vi "EncoderA(D13B)andLoadCell.vi"() -> ()   [LabVIEW 2021]
uses:
  BISS_1SL_interface_7.7.0/lv_interface/enum/BISS_InterfaceEnum.ctl
  BISS_1SL_interface_7.7.0/lv_interface/enum/BISS_InterfaceInfoEnum.ctl
  BISS_1SL_interface_7.7.0/lv_interface/enum/BISS_ComParamEnum.ctl
  BISS_1SL_interface_7.7.0/lv_interface/enum/BISS_FrameParamEnum.ctl
  BISS_1SL_interface_7.7.0/lv_interface/enum/BISS_EdsParamEnum.ctl
  BISS_1SL_interface_7.7.0/lv_interface/enum/BISS_ErrorTypeEnum.ctl
  BISS_1SL_interface_7.7.0/lv_interface/dll_demo/BiSS Interface Demo Functions.ctl
  BISS_1SL_interface_7.7.0/lv_interface/BISS1SL_Interface.lvlib
panel:
  in  "Stop Button":bool
  in  "TabControl":T1(tab)
  in  "BISS_InterfaceInfoEnum":T2 format="0x%02x"
  out "BISS_InterfaceEnum":T3 format="0x%02x"
  in  "BISS_InterfaceEnum":T3=enum."BISS_MB5U" format="0x%02x"
  in  "Close":bool caption="BiSS_Close"
  in  "Get Interface":bool caption="BiSS_GetInterface"
  in  "Set Interface":bool caption="BiSS_SetInterface"
  in  "Open":bool caption="BiSS_Open"
  in  "pcInterfaceOption":string="D13B"
  in  "Get Interface Info":bool caption="BiSS_GetInterfaceInfo"
  out "pcInterfaceInfo":string
  in  "Write Master Params":bool caption="BiSS_WriteMasterParams"
  in  "pcFilename":path
  in  "Load DLL Config":bool caption="BiSS_LoadDLLConfig"
  in  "pcFilename 2":path=path "C:/Users/TSSW/Documents/Kenneth Feb/BISS Test Vi/BiSS_config.cfg"
  in  "Save DLL Config":bool caption="BiSS_SaveDLLConfig"
  in  "Get Slave Label":bool caption="BiSS_GetSlaveLabel"
  in  "ulSlave 2":u32 format="%.0x"
  out "pcCompleteLabel 2":string
  out "pcSlaveLabel 2":string
  out "pcManufacturerLabel 2":string
  in  "Set FTDI Freq":bool caption="BiSS_SetFTDIFreq"
  in  "ulFreqL":u32=4 format="%0x"
  in  "ulFreqH":u32=4 format="%0x"
  out "Force vs Displacement":cluster{"X":dbl, "Y":dbl}[](graph)
  out "Displacement vs Time":waveform(sgl)(graph)
  out "pulValues":u64[](array[numeric]) format="%.0x"
  in  "ulCycleCount":u32 format="%.0x"
  in  "ulContentIndex":u32 format="%.0x"
  in  "ulDataChannel":u32 format="%.0x"
  in  "Get SCD Frame Content Ex":bool caption="BiSS_GetScdFrameContentEx"
  in  "Read SCD Frames":bool caption="BiSS_ReadScdFrames"
  in  "ulCycleCnt":u32=1 format="%.0x"
  out "pulDataScdH":u32[](array[numeric]) format="%.0x"
  out "pulDataScdL":sgl[](array[numeric]) format="%#_8g mm"
  out "pulStatus":u32[](array[numeric]) format="%.0x"
  out "pulTimestamp":u32[](array[numeric]) format="%.0x"
  in  "Get SCD Frame":bool caption="BiSS_GetScdFrame"
  in  "ulFrameIndex":u32 format="%.0x"
  out "pulDataScdH":u32[](array[numeric]) format="%.0x"
  out "pulDataScdL":u32[](array[numeric]) format="%.0x"
  out "pulStatus":u32 format="%.0x"
  out "pulTimestamp":u32 format="%.0x"
  in  "ulDataChannel":u32 format="%.0x"
  in  "Get SCD Frame Ex":bool caption="BiSS_GetScdFrameEx"
  in  "ulCycleCount":u32 format="%.0x"
  out "pulTimestamp":u32[](array[numeric]) format="%.0x"
  out "pulDataScdH":u32[](array[numeric]) format="%.0x"
  out "pulDataScdL":u32[](array[numeric]) format="%.0x"
  out "pulStatus":u32[](array[numeric]) format="%.0x"
  in  "Get SCD Frame Content":bool caption="BiSS_GetScdFrameContent"
  in  "ulDataChannel":u32 format="%.0x"
  in  "ulContentIndex":u32 format="%.0x"
  out "pulValues":u32[](array[numeric]) format="%.0x"
  in  "ulCycleCount":u32 format="%.0x"
  in  "stop":bool
  out "Loop Time [ms]":u32
  in  "Update Time [ms]":u32=1000
  out "error out 2":errorcluster
  in  "data":dbl[](array[numeric])=[0.0] min=0.0 max=7.0 step=0.1
  out "Load Cells Display":string
  out "error out":errorcluster
  out "Load A [kN]":dbl(slide) scale=-100.0..100.0
  out "Load B [kN]":dbl(slide) scale=-60.0..60.0
  out "Load A vs Time":waveform(dbl)(graph)
  out "BISS_ErrorTypeEnum":T4 format="0x%02x"
  in  "Get DLL Version":bool caption="BiSS_GetDLLVersion"
  out "pulDllVersion":u32[](array[numeric]) format="%.0x"
  in  "Calculate CRC":bool caption="BiSS_CalculateCRC"
  in  "ulCrcPoly":u32 format="%.0x"
  in  "pulData":u32[](array[numeric]) format="%.0x"
  in  "ulByteCount":u32 format="%.0x"
  out "pulCheckSum":u32 format="%.0x"
  in  "Calculate CRC Ex":bool caption="BiSS_CalculateCRCEx"
  out "pulCheckSum":u32 format="%.0x"
  in  "ulByteCount":u32 format="%.0x"
  in  "pulData":u32[](array[numeric]) format="%.0x"
  in  "ulCrcPoly":u32 format="%.0x"
  in  "ulCRCStartValue":u32 format="%.0x"
  in  "Get Last Error":bool caption="BiSS_GetLastError"
  out "pulLastError":u32 format="%0x"
  out "pcErrorText":string
  in  "Get MB3U Pins":bool caption="BiSS_GetMB3UPins"
  out "pulDir":u32 format="%.0x"
  out "pulValue":u32 format="%.0x"
  in  "ulDir":u32 format="%.0x"
  in  "Set MB3U Pins":bool caption="BiSS_SetMB3UPins"
  in  "ulValue":u32 format="%.0x"
  in  "Set Slave Label":bool caption="BiSS_SetSlaveLabel"
  in  "ulSlave":u32 format="%.0x"
  in  "pcSlaveLabel":string
  in  "pcManufacturerLabel":string
  in  "pcCompleteLabel":string
  in  "Set SCD Content Labels":bool caption="BiSS_SetScdContentLabels"
  in  "ulDataChannel":u32 format="%.0x"
  in  "ulContentIndex":u32 format="%.0x"
  in  "pcScdContentLabel":string
  in  "pcScdContentUnit":string
  in  "Get SCD Content Labels":bool caption="BiSS_GetScdContentLabels"
  in  "ulDataChannel":u32 format="%.0x"
  in  "ulContentIndex":u32 format="%.0x"
  out "pcSCDContentLabel":string
  out "pcSCDContentUnit":string
  in  "BISS_FrameParamEnum":T5 format="0x%02x"
  in  "BISS_FrameParamEnum":T5 format="0x%02x"
  in  "BISS_ComParamEnum":T6 format="0x%02x"
  in  "BISS_ComParamEnum":T6 format="0x%02x"
  in  "pcFilename":path
  in  "Set Com Param":bool caption="BiSS_SetComParam"
  in  "Auto Detection":bool caption="BiSS_Autodetection"
  in  "ulWriteMasterParams":u32 format="%.0x"
  out "pulSlaveCount":u32 format="%.0x"
  in  "ulValue":u32 format="%.0x"
  in  "Get Com Param":bool caption="BiSS_GetComParam"
  out "pulValue":u32 format="%.0x"
  in  "Set Frame Param":bool caption="BiSS_FrameParamEnum"
  in  "ulDataChannel":u32 format="%.0x"
  in  "ulValue":u32 format="%.0x"
  in  "Get Frame Param":bool caption="BiSS_GetFrameParam"
  out "pulValue":u32 format="%.0x"
  in  "ulDataChannel":u32 format="%.0x"
  in  "Init BiSS Comm":bool caption="BiSS_InitBissComm"
  in  "Write Slave Register":bool caption="BiSS_WriteSlaveRegister"
  in  "ulProtocol":u32 format="%.0x"
  in  "ulSlaveId":u32 format="%.0x"
  in  "ulRegisterAddress":u32 format="%.0x"
  in  "pulRegisterContent":u32[](array[numeric]) format="%.0x"
  in  "pulNumberOfBytes":u32 format="%.0x"
  in  "Read Slave Register":bool caption="BiSS_ReadSlaveRegister"
  in  "ulProtocol":u32 format="%.0x"
  in  "ulSlaveId":u32 format="%.0x"
  in  "ulRegisterAddress":u32 format="%.0x"
  in  "pulNumberOfBytes":u32 format="%.0x"
  out "pulRegisterContent":u32[](array[numeric]) format="%.0x"
  in  "Read SCD":bool caption="BiSS_ReadSCD"
  in  "ulStartControlFrame":u32 format="%.0x"
  out "pulScdValid":u32 format="%.0x"
  out "pulControlFrameEnd":u32 format="%.0x"
  out "pulDataScdH":u32[](array[numeric]) format="%.0x"
  out "pulDataScdL":u32[](array[numeric]) format="%.0x"
  in  "ulIds":u32 format="%.0x"
  in  "ulCmd":u32 format="%.0x"
  in  "Send Command":bool caption="BiSS_SendCommand"
  in  "Get SCD Content":bool caption="BiSS_GetScdContent"
  in  "ulDataChannel":u32 format="%.0x"
  out "pulScdContentValues":u32[](array[numeric]) format="%.0x"
  in  "Get SCD Content Ex":bool caption="BiSS_GetScdContentEx"
  in  "ulDataChannel":u32 format="%.0x"
  out "pulScdContentValues":u64[](array[numeric]) format="%.0x"
  in  "Set SCD Content Params":bool caption="BiSS_SetScdContentParams"
  in  "ulDataChannel":u32 format="%.0x"
  in  "ulContentIndex":u32 format="%.0x"
  in  "pScdContentItems":T7 {"lOffset" format="%.0x"; "ulResolution" format="%.0x"; "ulDataLength" format="%.0x"; "ulZero" format="%.0x"}
  in  "Get SCD Content Params":bool caption="BiSS_GetScdContentParams"
  in  "ulDataChannel":u32 format="%.0x"
  in  "ulContentIndex":u32 format="%.0x"
  out "pScdContentItems":T7 {"ulZero" format="%.0x"; "ulDataLength" format="%.0x"; "ulResolution" format="%.0x"; "lOffset" format="%.0x"}
  in  "BISS_EdsParamEnum":T8 format="0x%02x"
  in  "BISS_EdsParamEnum":T8 format="0x%02x"
  in  "Set EDS Param":bool caption="BiSS_SetEdsParam"
  in  "ulValue":u32 format="%.0x"
  out "pulValue":u32 format="%.0x"
  in  "Get EDS Param":bool caption="BiSS_GetEdsParam"
  in  "Set EDS Register":bool caption="BiSS_SetEdsRegister"
  in  "ulAdr":u32 format="%.0x"
  in  "ulValue":u32 format="%.0x"
  in  "Get EDS Register":bool caption="BiSS_GetEdsRegister"
  in  "ulAdr":u32 format="%.0x"
  out "pulValue":u32 format="%.0x"
  in  "Read EDS Params":bool caption="BiSS_ReadEdsParams"
  in  "ulSlaveId":u32 format="%.0x"
  in  "Write EDS Params":bool caption="BiSS_WriteEdsParams"
  in  "ulSlaveId":u32 format="%.0x"
  in  "pcFilename":path
  in  "Write Master Register":bool caption="BiSS_ WriteMasterRegister"
  in  "ulRegisterAddress":u32 format="%.0x"
  in  "ulRegisterContent":u32 format="%.0x"
  in  "Read Master Register":bool caption="BiSS_ ReadMasterRegister"
  in  "ulRegisterAddress":u32 format="%.0x"
  out "pulRegisterContent":u32 format="%.0x"
  in  "Get Master Register":bool caption="BiSS_ GetMasterRegister"
  in  "ulRegisterAddress":u32 format="%.0x"
  out "pulRegisterContent":u32 format="%.0x"
  in  "Save Master Config":bool caption="BiSS_ SaveMasterConfig"
  in  "pcFilename":path
  in  "Save Register":bool caption="BiSS_ SaveRegister"
  in  "pcFilename":path
  in  "ulStartAdr":u32 format="%.0x"
  in  "ulNumberOfBytes":u32 format="%.0x"
  in  "pulData":u32[](array[numeric]) format="%.0x"
  in  "Load Register":bool caption="BiSS_ LoadRegister"
  in  "ulStartAdr":u32 format="%.0x"
  in  "ulNumberOfBytes":u32 format="%.0x"
  out "pulData":u32[](array[numeric]) format="%.0x"
  # "BiSS Interface Library Demo"
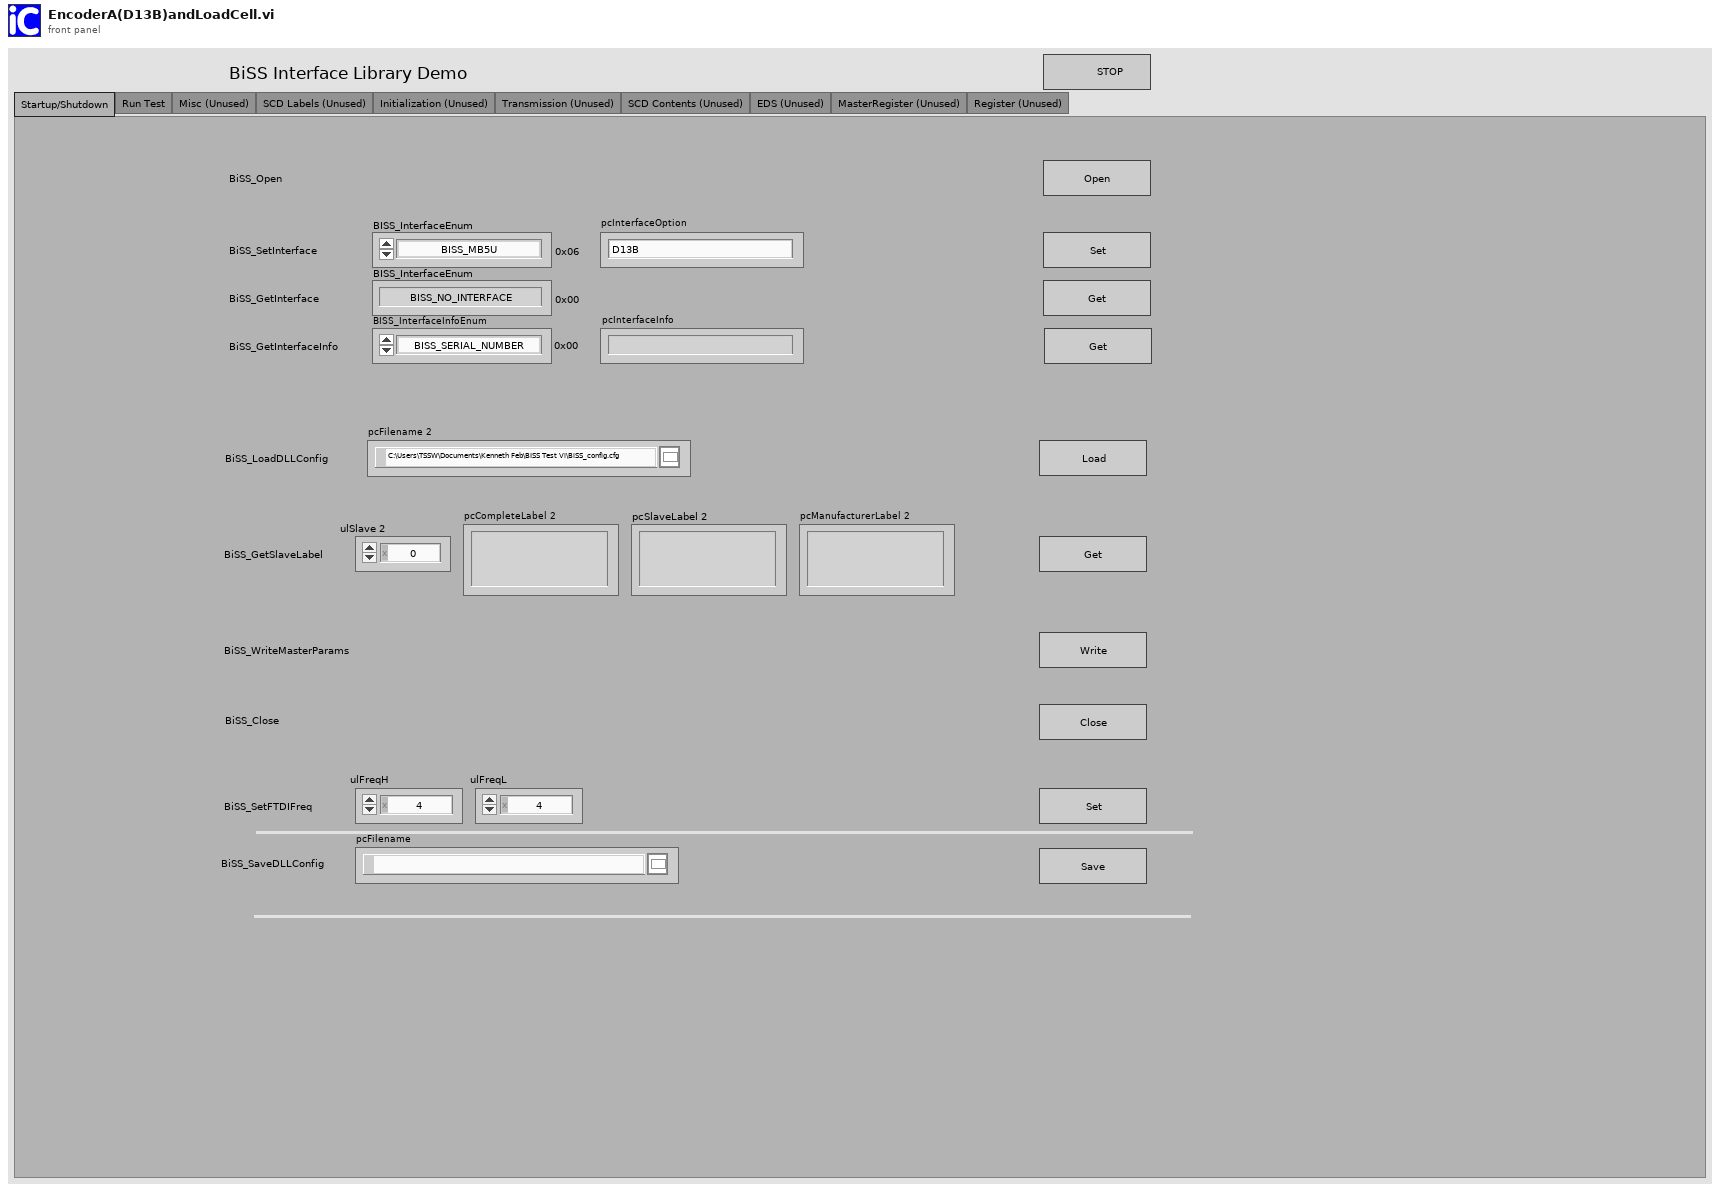
[diagram p1: front panel]
types:
  T1 = enum32{"Startup/Shutdown", "Run Test", "Misc (Unused)", "SCD Labels (Unused)", "Initialization (Unused)", "Transmission (Unused)", "SCD Contents (Unused)", "EDS (Unused)", "MasterRegister (Unused)", "Register (Unused)"}
  T2 = typedef "BISS1SL_Interface.lvlib/BISS_InterfaceInfoEnum.ctl" = enum32{"BISS_SERIAL_NUMBER", "BISS_DRIVER_VERSION"}
  T3 = typedef "BISS1SL_Interface.lvlib/BISS_InterfaceEnum.ctl" = enum32{"BISS_NO_INTERFACE", "BISS_MB3D_INT", "BISS_MB3D_MOT", "BISS_MB3A", "BISS_MB3U", "BISS_MB4U", "BISS_MB5U", "BISS_MB3U_SPI"}
  T4 = typedef "BISS1SL_Interface.lvlib/BISS_ErrorTypeEnum.ctl" = enum32{"BISS_NONE", "BISS_HINT", "BISS_WARNING", "BISS_PROGRAMMING_ERROR", "BISS_OPERATING_ERROR", "BISS_COMMUNICATION_ERROR"}
  T5 = typedef "BISS1SL_Interface.lvlib/BISS_FrameParamEnum.ctl" = enum32{"BISS_SCD_LENGTH", "BISS_SCD_CRC_POLY", "BISS_SCD_CRC_INVERT", "BISS_SCD_CONTENT_COUNT", "BISS_RESERVED", "BISS_SLAVEID", "BISS_IDCOUNT", "BISS_CRCS", "BISS_GRAYS", "BISS_GRAY_MSB", "BISS_GRAY_LSB", "BISS_CRC_CLOSING_VALUE"}
  T6 = typedef "BISS1SL_Interface.lvlib/BISS_ComParamEnum.ctl" = enum32{"BISS_MASTER_VERSION", "BISS_MASTER_REVISION", "BISS_PROTOCOL", "BISS_CLKENI", "BISS_FREQ_SCD", "BISS_FREQ_REG", "BISS_FREQ_AGS", "BISS_SLAVE_ID", "BISS_REGISTER_ADDRESS", "BISS_WNR", "BISS_REGISTER_VALUE", "BISS_SSIWRITE", "BISS_SSIWRITE_TIMEOUT", "BISS_MAX_DATACH_CNT", "BISS_MAX_REG_CNT", "BISS_EN_MO", "BISS_FREQ_AGS_REG", "BISS_EDS_BANK", "BISS_DISABLE_TIMEOUT", "BISS_ENABLE_TTL", "BISS_NUMBER_OF_DATA_CHANNELS", "BISS_SSIWRITE_DL", "BISS_SLAVELOC"}
  T7 = cluster{"ulZero":u32, "ulDataLength":u32, "ulResolution":u32, "lOffset":i32}
  T8 = typedef "BISS1SL_Interface.lvlib/BISS_EdsParamEnum.ctl" = enum32{"BISS_EDS_EDS_VER", "BISS_EDS_EDS_LEN", "BISS_EDS_USR_STA", "BISS_EDS_USR_END", "BISS_EDS_TMA", "BISS_EDS_TO_MIN", "BISS_EDS_TO_MAX", "BISS_EDS_TOS_MIN", "BISS_EDS_TOS_MAX", "BISS_EDS_TCLK_MIN", "BISS_EDS_TCLK_MAX", "BISS_EDS_TCYC", "BISS_EDS_TBUSY_S", "BISS_EDS_BUSY_S", "BISS_EDS_PON_DLY", "BISS_EDS_DC_NUM", "BISS_EDS_SL_NUM", "BISS_EDS_SL_OFF", "BISS_EDS_BANK1", "BISS_EDS_DLEN1", "BISS_EDS_FORMAT1_STOP", "BISS_EDS_FORMAT1_ALIGN", "BISS_EDS_FORMAT1_TYPE", "BISS_EDS_CPOLY1", "BISS_EDS_BANK2", "BISS_EDS_DLEN2", "BISS_EDS_FORMAT2_STOP", "BISS_EDS_FORMAT2_ALIGN", "BISS_EDS_FORMAT2_TYPE", "BISS_EDS_CPOLY2", "BISS_EDS_BANK3", "BISS_EDS_DLEN3", "BISS_EDS_FORMAT3_STOP", "BISS_EDS_FORMAT3_ALIGN", "BISS_EDS_FORMAT3_TYPE", "BISS_EDS_CPOLY3", "BISS_EDS_BANK4", "BISS_EDS_DLEN4", "BISS_EDS_FORMAT4_STOP", "BISS_EDS_FORMAT4_ALIGN", "BISS_EDS_FORMAT4_TYPE", "BISS_EDS_CPOLY4", "BISS_EDS_BANK5", "BISS_EDS_DLEN5", "BISS_EDS_FORMAT5_STOP", "BISS_EDS_FORMAT5_ALIGN", "BISS_EDS_FORMAT5_TYPE", "BISS_EDS_CPOLY5", "BISS_EDS_BANK6", "BISS_EDS_DLEN6", "BISS_EDS_FORMAT6_STOP", "BISS_EDS_FORMAT6_ALIGN", "BISS_EDS_FORMAT6_TYPE", "BISS_EDS_CPOLY6", "BISS_EDS_BANK7", "BISS_EDS_DLEN7", "BISS_EDS_FORMAT7_STOP", "BISS_EDS_FORMAT7_ALIGN", "BISS_EDS_FORMAT7_TYPE", "BISS_EDS_CPOLY7", "BISS_EDS_BANK8", "BISS_EDS_DLEN8", "BISS_EDS_FORMAT8_STOP", "BISS_EDS_FORMAT8_ALIGN", "BISS_EDS_FORMAT8_TYPE", "BISS_EDS_CPOLY8", "BISS_EDS_BC_OFF", "BISS_EDS_BP_VER", "BISS_EDS_BP_LEN", "BISS_EDS_BP_ID", "BISS_EDS_FB1", "BISS_EDS_FB2", "BISS_EDS_PON_PDL", "BISS_EDS_EN_TYP", "BISS_EDS_POS_NUM", "BISS_EDS_MT_LEN", "BISS_EDS_MT_FMT", "BISS_EDS_CO_LEN", "BISS_EDS_CO_FMT", "BISS_EDS_FI_LEN", "BISS_EDS_FI_FMT", "BISS_EDS_MT_CNT", "BISS_EDS_SIP_CNT", "BISS_EDS_SIP_RES", "BISS_EDS_CPOLY", "BISS_EDS_CSTART", "BISS_EDS_ABS_ACU", "BISS_EDS_REL_ACU", "BISS_EDS_SPD_ACU", "BISS_EDS_HYST", "BISS_EDS_SPD_MAX", "BISS_EDS_ACC_MAX", "BISS_EDS_TMP_MIN", "BISS_EDS_TMP_MAX", "BISS_EDS_VLT_MIN", "BISS_EDS_VLT_MAX", "BISS_EDS_CUR_MAX"}
  T9 = typedef "BiSS Interface Demo Functions.ctl" = enum16{"Start Demo", "Open", "Close", "Set Interface", "Set Interface 2", "Get Interface", "Get Interface 2", "Get Interface Info", "Get Interface Info 2", "Auto Detection", "Set Com Param", "Get Com Param", "Set Frame Param", "Get Frame Param", "Write Master Params", "Set FTDI Freq", "Init BiSS Comm", "Write Slave Register", "Read Slave Register", "Read SCD", "Send Command", "Set Slave Label", "Get Slave Label", "Set SCD Content Labels", "Get SCD Content Labels", "Get SCD Content", "Get SCD Content Ex", "Set SCD Content Params", "Get SCD Content Params", "Read SCD Frames", "Get SCD Frame", "Get SCD Frame Ex", "Get SCD Frame Content", "Get SCD Frame Content Ex", "Set EDS Param", "Get EDS Param", "Set EDS Register", "Get EDS Register", "Read EDS Params", "Write EDS Params", "Get DLL Version", "Calculate CRC", "Calculate CRC Ex", "Save DLL Config", "Load DLL Config", "Get Last Error", "Get MB3U Pins", "Set MB3U Pins", "Write Master Register", "Read Master Register", "Get Master Register", "Save Master Config", "Save Register", "Load Register", "Stop Demo"}
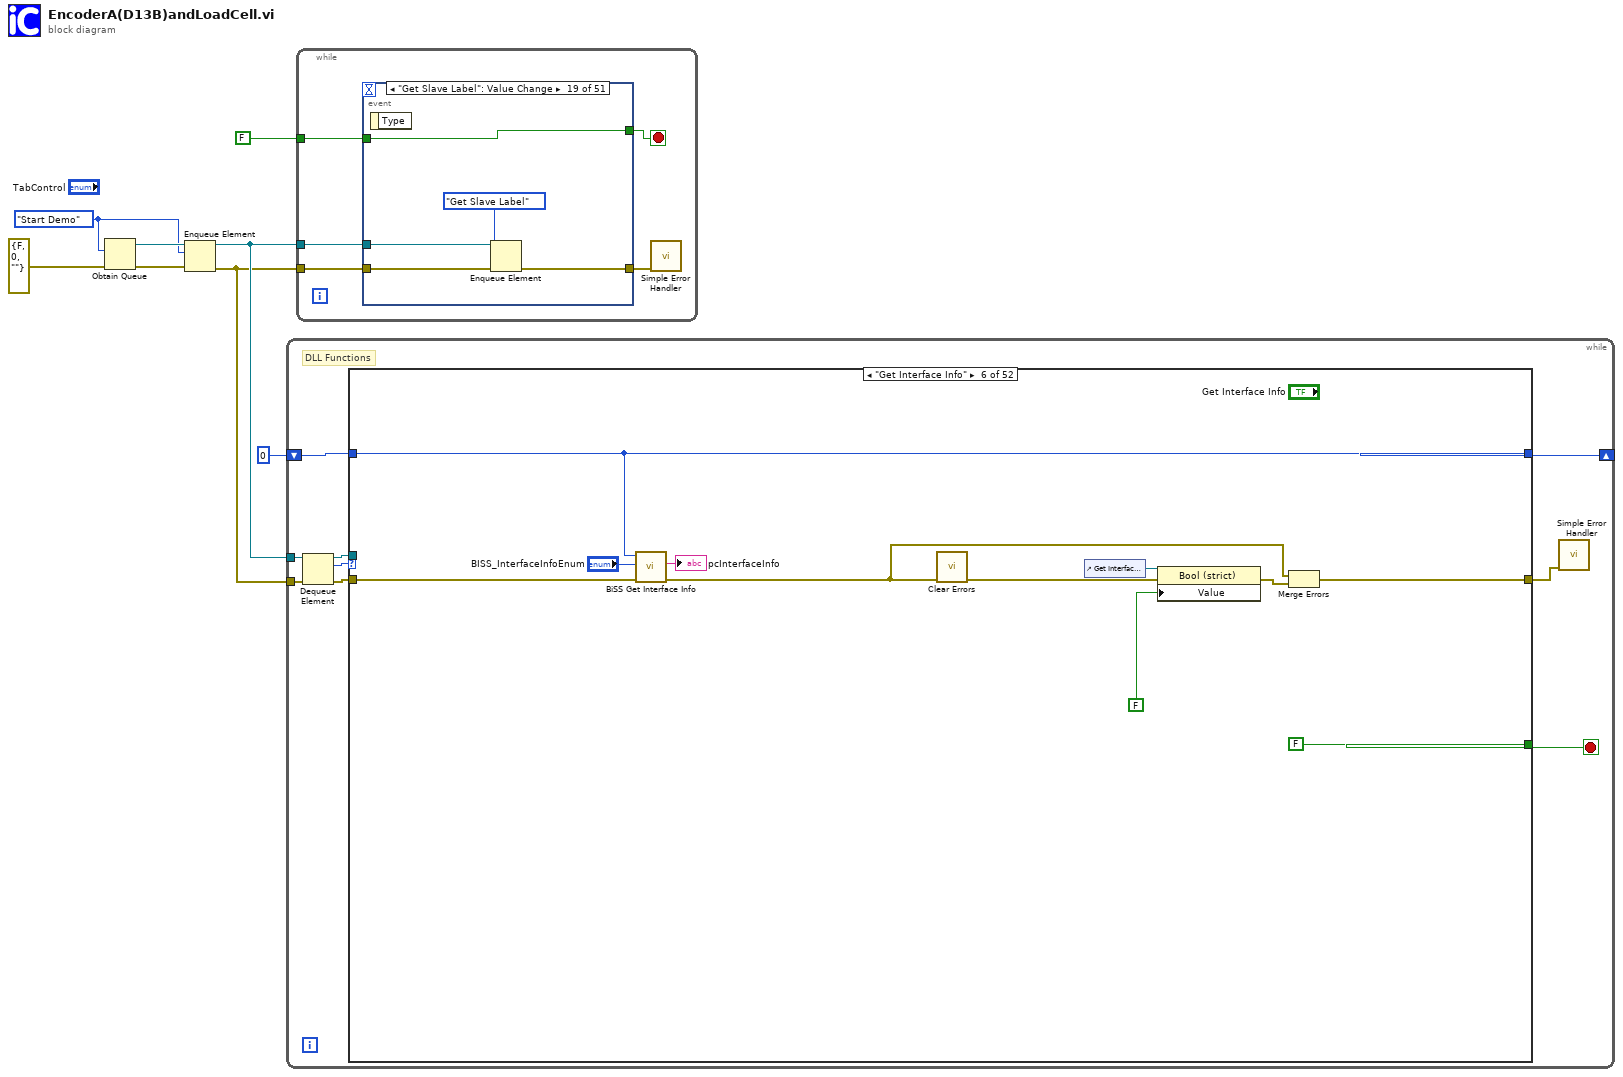
[diagram p0: block diagram]
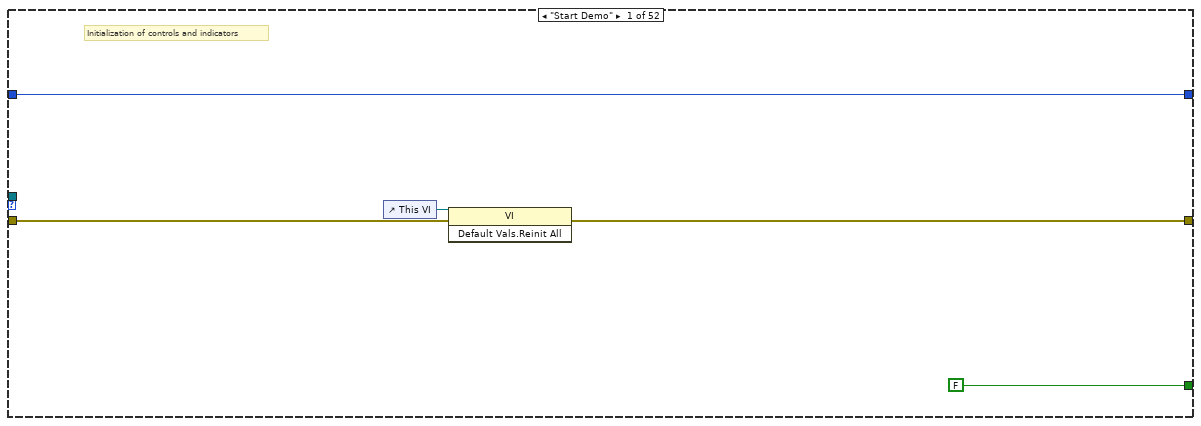
[diagram p2: hidden frame]
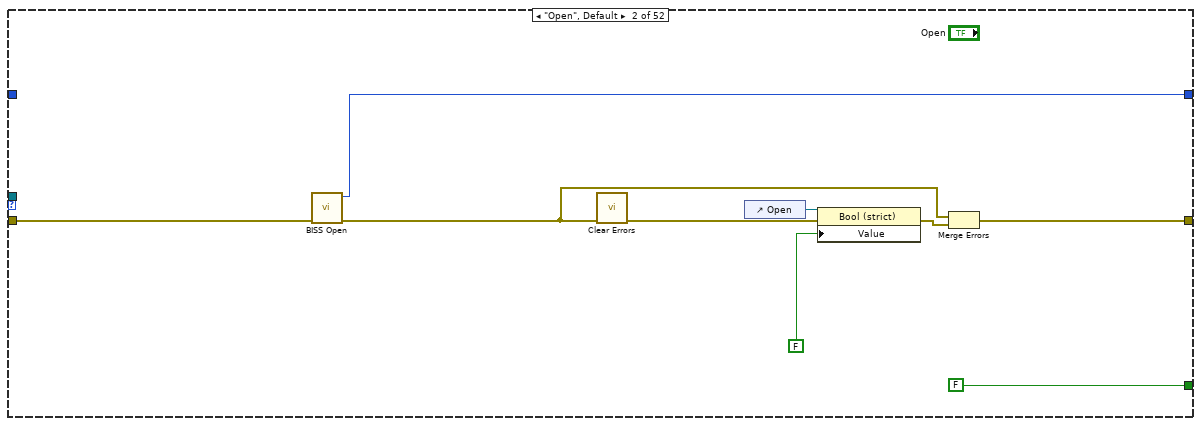
[diagram p3: hidden frame]
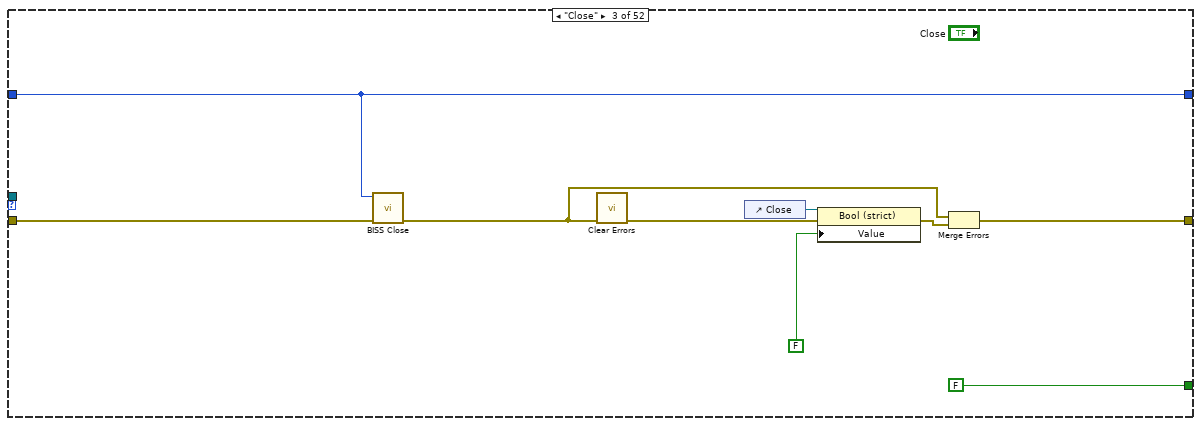
[diagram p4: hidden frame]
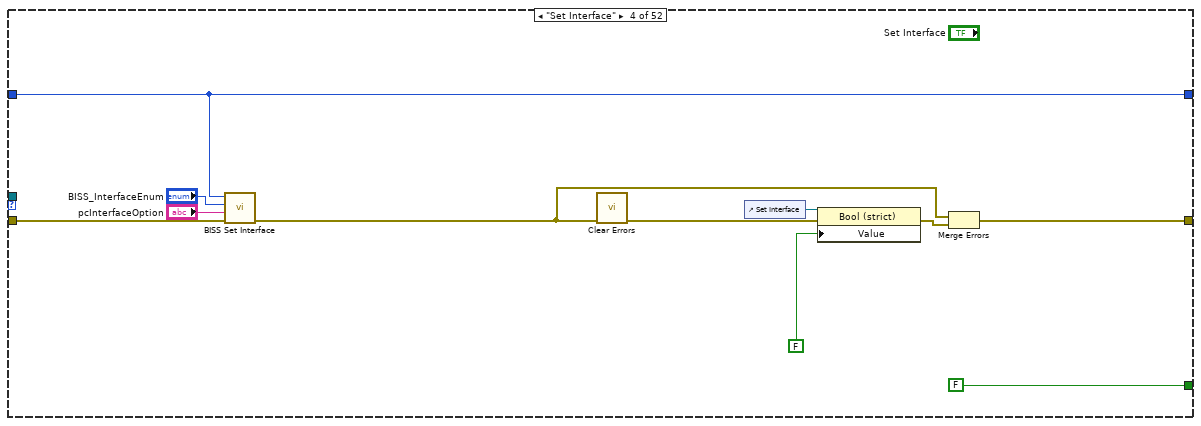
[diagram p5: hidden frame]
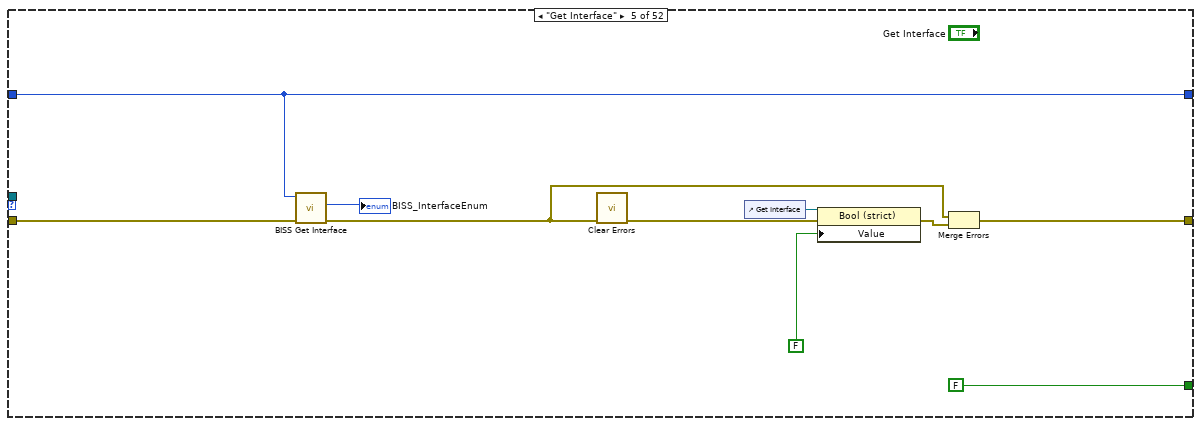
[diagram p6: hidden frame]
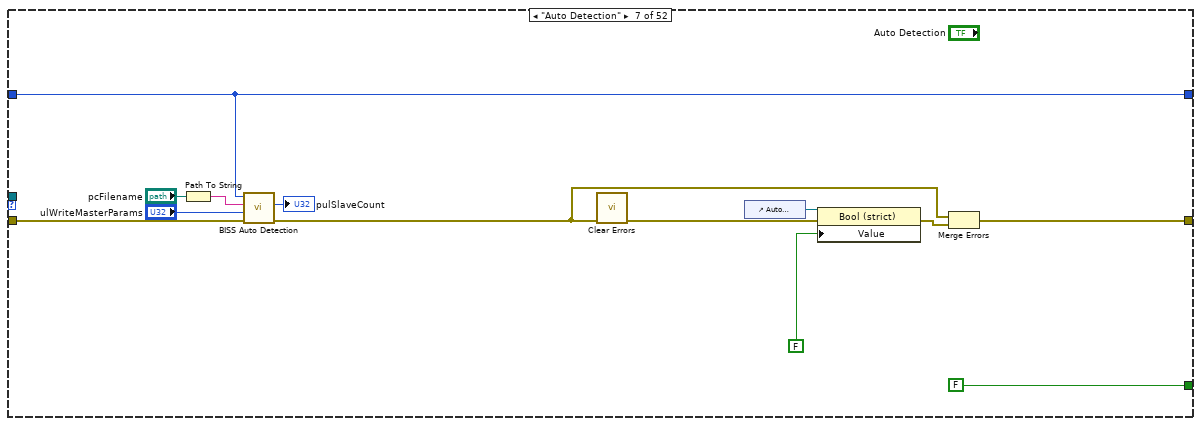
[diagram p7: hidden frame]
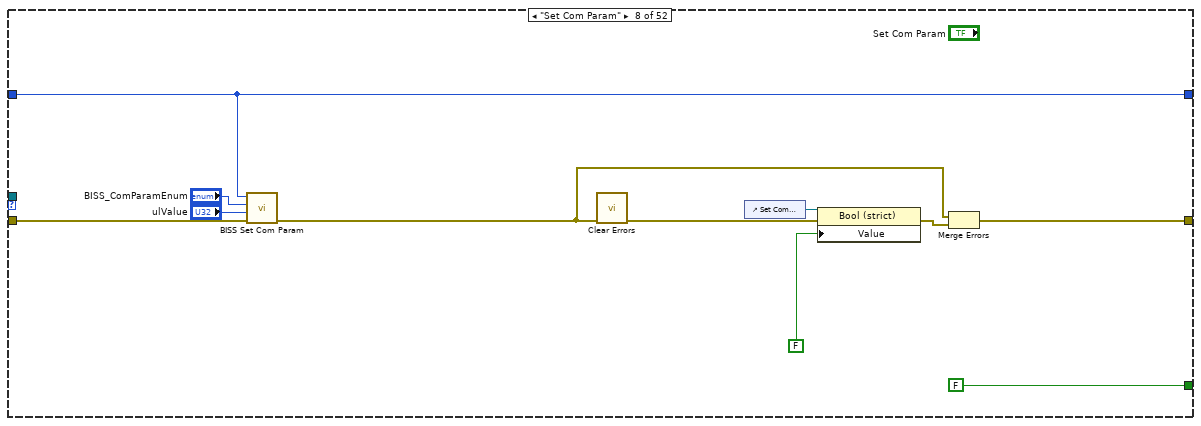
[diagram p8: hidden frame]
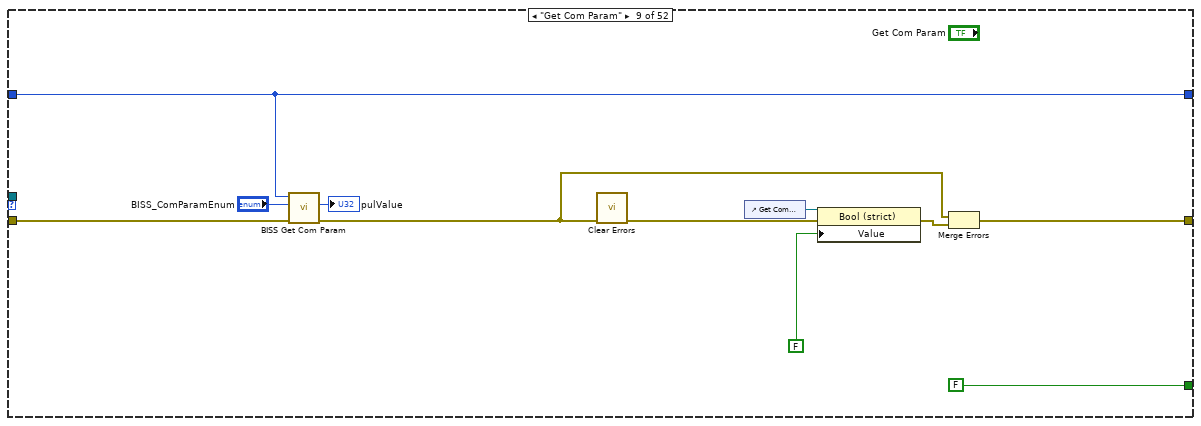
[diagram p9: hidden frame]
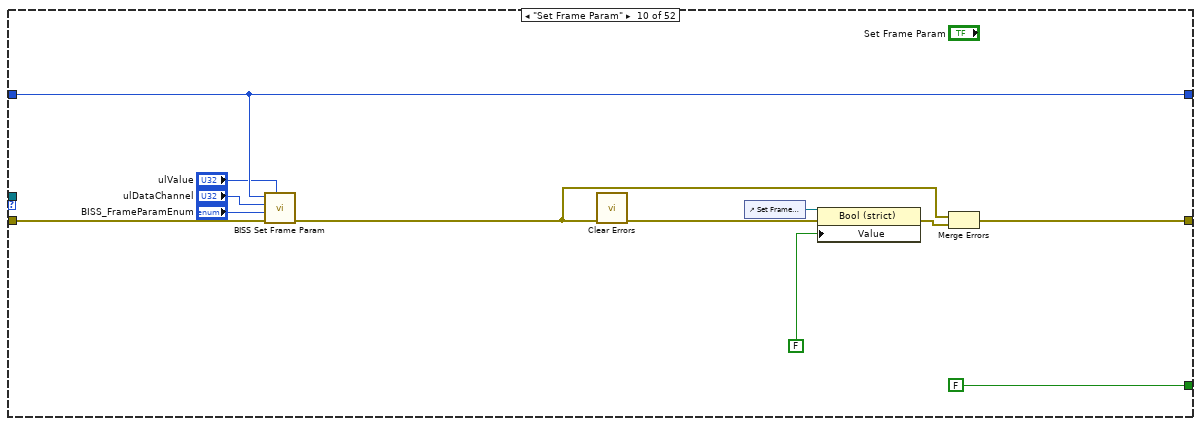
[diagram p10: hidden frame]
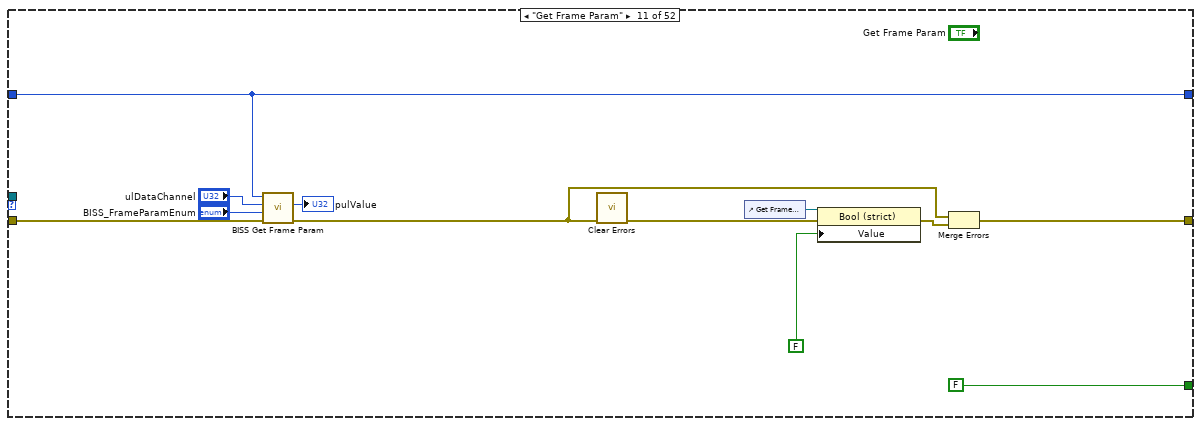
[diagram p11: hidden frame]
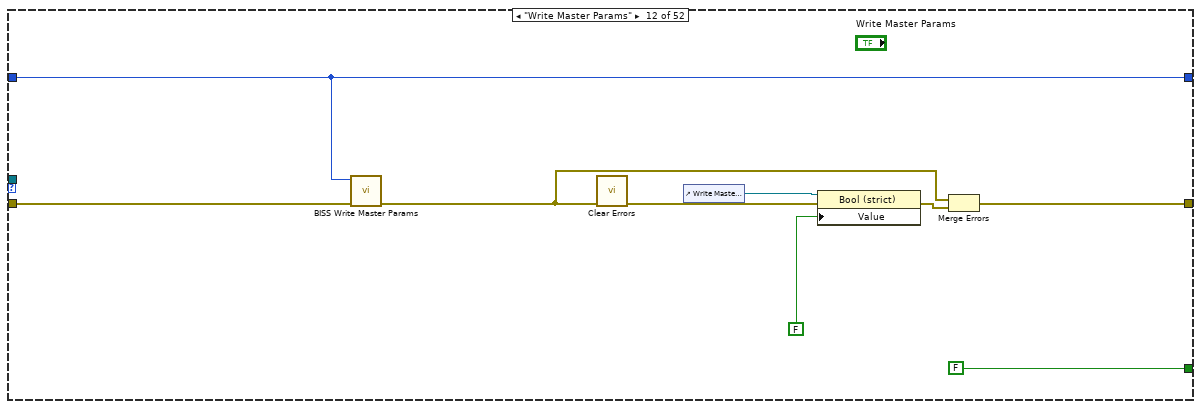
[diagram p12: hidden frame]
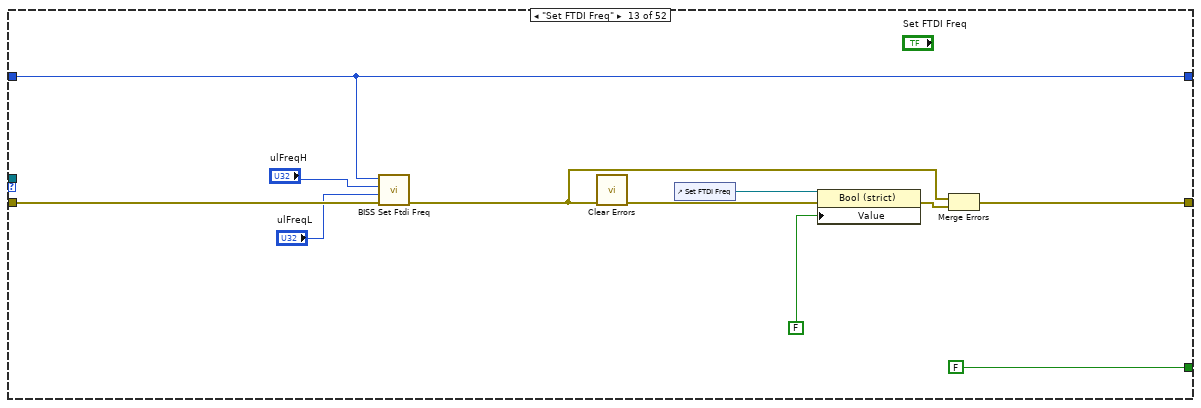
[diagram p13: hidden frame]
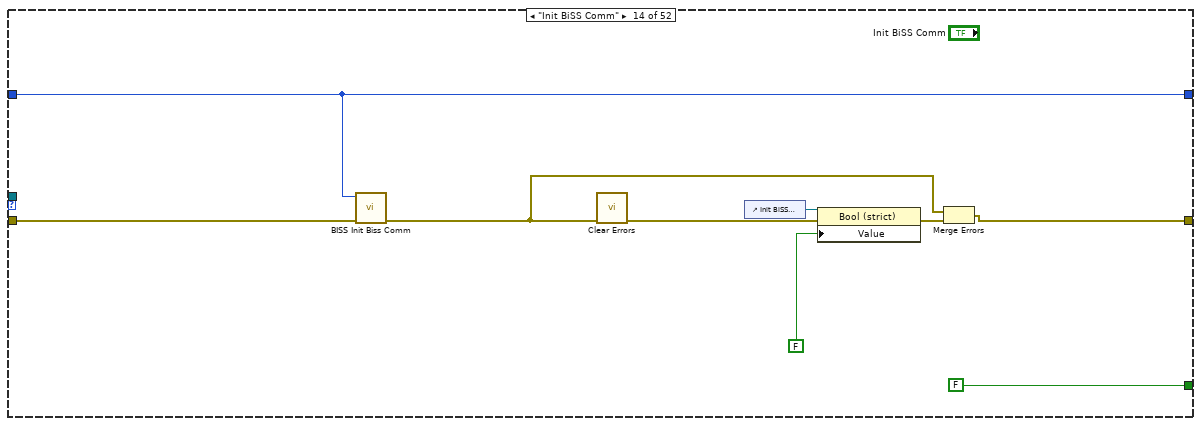
[diagram p14: hidden frame]
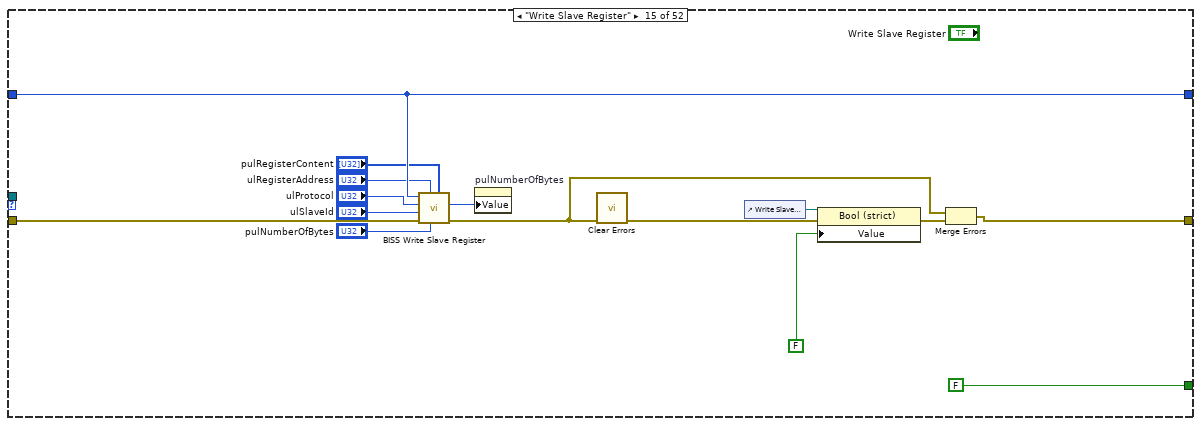
[diagram p15: hidden frame]
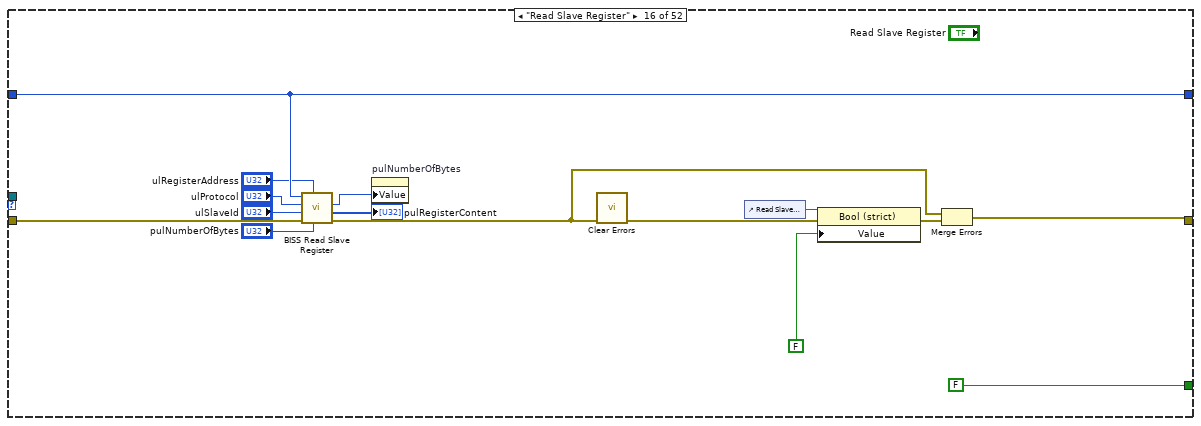
[diagram p16: hidden frame]
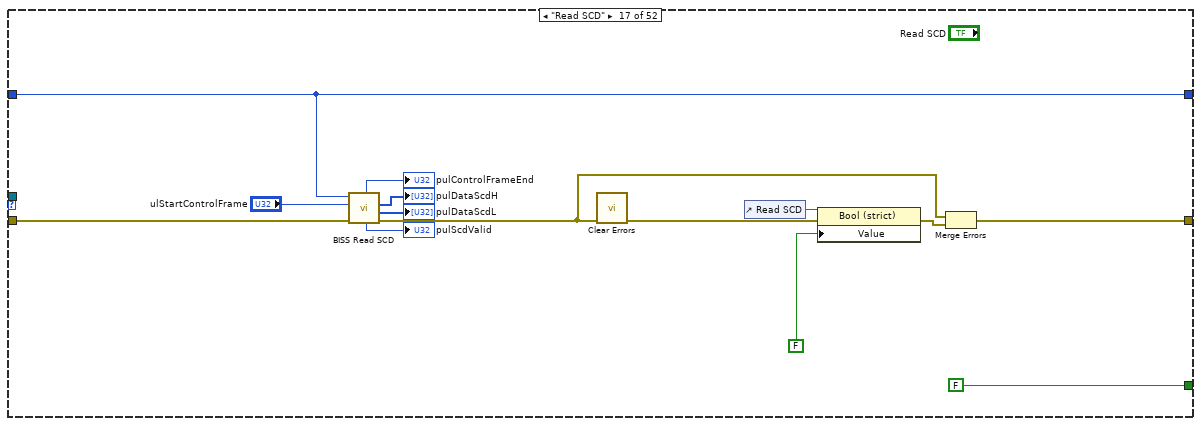
[diagram p17: hidden frame]
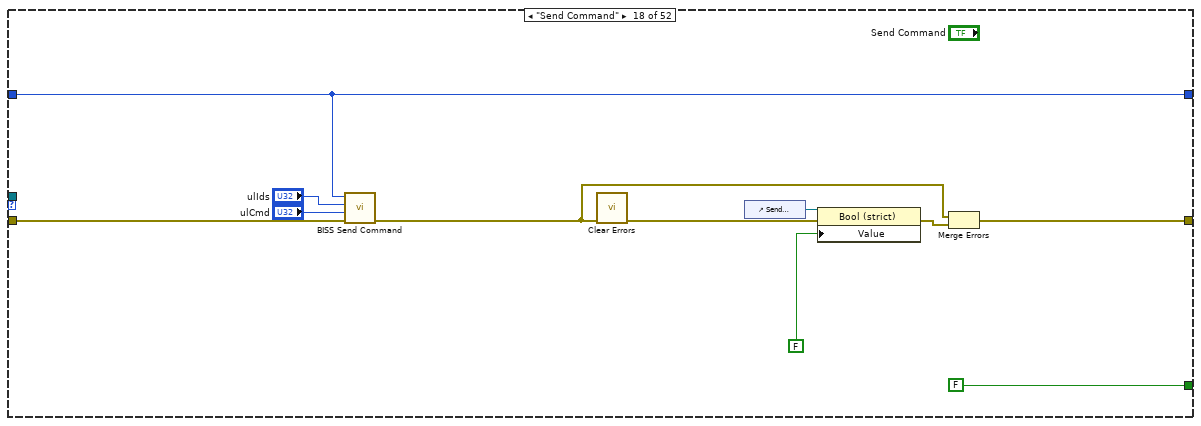
[diagram p18: hidden frame]
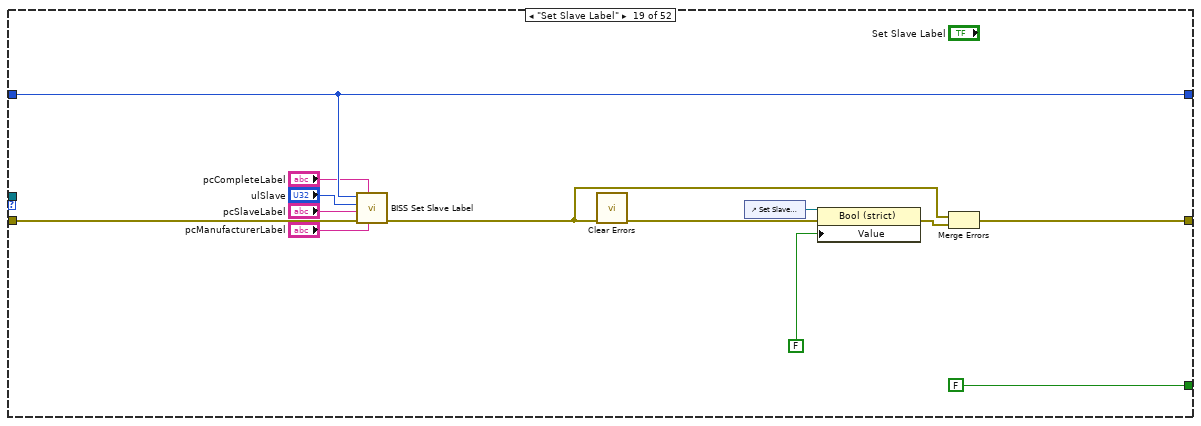
[diagram p19: hidden frame]
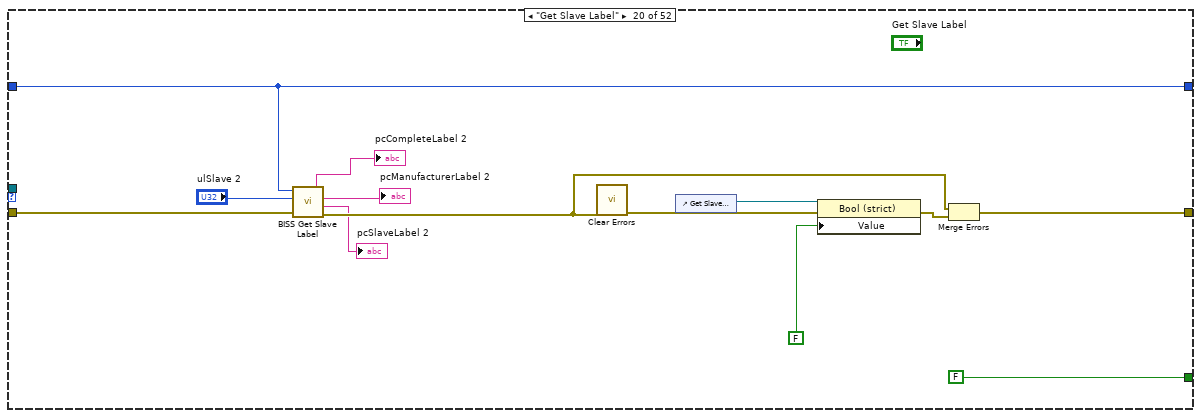
[diagram p20: hidden frame]
diagram:
  w2 = BiSS_Interface_Demo_Functions."Start Demo" ("Events")
  n1 = Obtain Queue(element data type=w2, error in (no error)=errorcluster {"status"=FALSE, "code"=0, "source"=""} ("error in")) -> (queue out=w7:refnum<queue>, error out=w8:errorcluster)  [unwired: 3 in, 1 out]
  n2 = Enqueue Element(queue=w7, element=w2, error in (no error)=w8) -> (queue out=w4:refnum<queue>, error out=w3:errorcluster)  [unwired: 1 in, 1 out]
  n3 = while {
    shift-right: [w15] -> _
    shift-left: u32 0 ("pulHTHandle") -> [w14]
    tunnel: w4 -> [w16]
    tunnel: w3 -> [w11]
    stop <- w12 stop-if-true
    # "DLL Functions"
    n4 = Dequeue Element(queue=w16, error in (no error)=w11) -> (queue out=w10:refnum<queue>, element=w17:T9, error out=w9:errorcluster)  [unwired: 1 in, 1 out]
    n5 = case shown="\"Get Interface Info\"" w17 {
      tunnel: [w18 w26 w36 w47 w57 w68 w82 w93 w104 w116 w128 w138 w147 w152 w170 w182 w200 w210 w224 w239 w250 w263 w274 w285 w297 w309 w318 w373 w388 w401 w407 w424 w435 w446 w457 w467 w477 w487 w500 w514 w526 w537 w548 w559 w570 w581 w592 w603 w614 w628 w642 w653] -> w13
      tunnel: [FALSE FALSE FALSE FALSE FALSE FALSE FALSE FALSE FALSE FALSE FALSE FALSE FALSE FALSE FALSE FALSE FALSE FALSE FALSE FALSE FALSE FALSE FALSE FALSE FALSE FALSE FALSE FALSE FALSE FALSE FALSE FALSE FALSE FALSE FALSE FALSE FALSE FALSE FALSE FALSE FALSE FALSE FALSE FALSE FALSE FALSE FALSE FALSE FALSE FALSE FALSE TRUE] -> w12
      tunnel: [w22 w23 w33 w44 w53 w64 w78 w89 w101 w112 w124 w133 w144 w155 w167 w185 w196 w209 w221 w236 w246 w259 w270 w281 w293 w305 w319 w371 w384 w397 w416 w421 w432 w445 w456 w464 w474 w486 w497 w511 w525 w536 w545 w556 w567 w578 w589 w600 w611 w625 w639 w657] -> w15
      tunnel: w14 -> [w22 _ w33 w44 w53 w64 w78 w89 w101 w112 w124 w133 w144 w155 w167 w185 w196 w209 w221 w236 w246 w259 w270 w281 w293 w305 w319 w371 w384 w397 w416 w421 w432 w445 w456 w464 w474 w486 w497 w511 w525 w536 w545 w556 w567 w578 w589 w600 w611 w625 w639 w657]
      tunnel: w10 -> [_ _ _ _ _ _ _ _ _ _ _ _ _ _ _ _ _ _ _ _ _ _ _ _ _ _ _ _ _ _ _ _ _ _ _ _ _ _ _ _ _ _ _ _ _ _ _ _ _ _ _ w654]
      tunnel: w9 -> [w19 w25 w34 w45 w55 w66 w79 w90 w100 w113 w125 w135 w146 w156 w169 w184 w198 w208 w222 w235 w248 w261 w272 w283 w295 w307 w320 w370 w386 w399 w417 w423 w434 w444 w455 w466 w476 w485 w499 w513 w524 w535 w547 w558 w569 w580 w591 w602 w613 w627 w641 w655]
      frame "Start Demo" {
        # "Initialization of controls and indicators"
        n6 = control-ref of="This VI"() -> (w20:refnum<vi>)
        n7 = invoke class="VI" method="Default Vals.Reinit All"(reference=w20, error in=w19) -> (error out=w18:errorcluster)  [unwired: 1 in, 2 out]
      }
      frame "Open", Default {
        n8 = call "BISS Open.vi"("Error In"=w25) -> ("Error Out"=w24:errorcluster, "pulBISSHandle"=w23:u32)  [unwired: 7 in, 2 out]
        n9 = call <vilib>:"Clear Errors.vi"("error in (no error)"=w24) -> ("error out"=w28:errorcluster)  [unwired: 5 in, 1 out]
        n10 = control-ref of="Open"() -> (w30:refnum<vi>)
        n11 = property class="Bool (strict)"(reference=w30, error in=w28, "Value"=FALSE) -> (error out=w27:errorcluster)  [unwired: 1 out]
        n12 = Merge Errors(w24, w27) -> (w26:errorcluster)
      }
      frame "Close" {
        n13 = call "BISS Close.vi"("Error In"=w34, "ulBISSHandle"=w33) -> ("Error Out"=w32:errorcluster)  [unwired: 7 in, 2 out]
        n14 = call <vilib>:"Clear Errors.vi"("error in (no error)"=w32) -> ("error out"=w35:errorcluster)  [unwired: 5 in, 1 out]
        n15 = control-ref of="Close"() -> (w38:refnum<vi>)
        n16 = property class="Bool (strict)"(reference=w38, error in=w35, "Value"=FALSE) -> (error out=w37:errorcluster)  [unwired: 1 out]
        n17 = Merge Errors(w32, w37) -> (w36:errorcluster)
      }
      frame "Set Interface" {
        n18 = call "BISS Set Interface.vi"("Error In"=w45, "pcInterfaceOption"="pcInterfaceOption", "ulInterface"="BISS_InterfaceEnum", "ulBISSHandle"=w44) -> ("Error Out"=w43:errorcluster)  [unwired: 5 in, 2 out]
        n19 = call <vilib>:"Clear Errors.vi"("error in (no error)"=w43) -> ("error out"=w48:errorcluster)  [unwired: 5 in, 1 out]
        n20 = control-ref of="Set Interface"() -> (w49:refnum<vi>)
        n21 = property class="Bool (strict)"(reference=w49, error in=w48, "Value"=FALSE) -> (error out=w46:errorcluster)  [unwired: 1 out]
        n22 = Merge Errors(w43, w46) -> (w47:errorcluster)
      }
      frame "Get Interface" {
        n23 = call "BISS Get Interface.vi"("Error In"=w55, "ulBISSHandle"=w53) -> ("Error Out"=w54:errorcluster, "pulInterface"=→"BISS_InterfaceEnum":u32)  [unwired: 6 in, 2 out]
        n24 = call <vilib>:"Clear Errors.vi"("error in (no error)"=w54) -> ("error out"=w56:errorcluster)  [unwired: 5 in, 1 out]
        n25 = control-ref of="Get Interface"() -> (w59:refnum<vi>)
        n26 = property class="Bool (strict)"(reference=w59, error in=w56, "Value"=FALSE) -> (error out=w58:errorcluster)  [unwired: 1 out]
        n27 = Merge Errors(w54, w58) -> (w57:errorcluster)
      }
      frame "Get Interface Info" {
        n28 = call "BiSS Get Interface Info.vi"("Error In"=w66, "ulIndex"="BISS_InterfaceInfoEnum", "ulBISSHandle"=w64) -> ("Error Out"=w65:errorcluster, "pcInterfaceInfo"=→"pcInterfaceInfo":string)  [unwired: 5 in, 2 out]
        n29 = call <vilib>:"Clear Errors.vi"("error in (no error)"=w65) -> ("error out"=w67:errorcluster)  [unwired: 5 in, 1 out]
        n30 = control-ref of="Get Interface Info"() -> (w70:refnum<vi>)
        n31 = property class="Bool (strict)"(reference=w70, error in=w67, "Value"=FALSE) -> (error out=w69:errorcluster)  [unwired: 1 out]
        n32 = Merge Errors(w65, w69) -> (w68:errorcluster)
      }
      frame "Auto Detection" {
        n33 = Path To String(path="pcFilename") -> (string=w76:string)
        n34 = call "BISS Auto Detection.vi"("Error In"=w79, "ulWriteMasterParams"="ulWriteMasterParams", "pcFilename"=w76, "ulBISSHandle"=w78) -> ("Error Out"=w73:errorcluster, "pulSlaveCount"=→"pulSlaveCount":u32)  [unwired: 4 in, 2 out]
        n35 = call <vilib>:"Clear Errors.vi"("error in (no error)"=w73) -> ("error out"=w80:errorcluster)  [unwired: 5 in, 1 out]
        n36 = control-ref of="Auto Detection"() -> (w83:refnum<vi>)
        n37 = property class="Bool (strict)"(reference=w83, error in=w80, "Value"=FALSE) -> (error out=w81:errorcluster)  [unwired: 1 out]
        n38 = Merge Errors(w73, w81) -> (w82:errorcluster)
      }
      frame "Set Com Param" {
        n39 = call "BISS Set Com Param.vi"("Error In"=w90, "ulValue"="ulValue", "ulParam"="BISS_ComParamEnum", "ulBISSHandle"=w89) -> ("Error Out"=w88:errorcluster)  [unwired: 5 in, 2 out]
        n40 = call <vilib>:"Clear Errors.vi"("error in (no error)"=w88) -> ("error out"=w91:errorcluster)  [unwired: 5 in, 1 out]
        n41 = control-ref of="Set Com Param"() -> (w94:refnum<vi>)
        n42 = property class="Bool (strict)"(reference=w94, error in=w91, "Value"=FALSE) -> (error out=w92:errorcluster)  [unwired: 1 out]
        n43 = Merge Errors(w88, w92) -> (w93:errorcluster)
      }
      frame "Get Com Param" {
        n44 = call "BISS Get Com Param.vi"("Error In"=w100, "ulParam"="BISS_ComParamEnum", "ulBISSHandle"=w101) -> ("Error Out"=w99:errorcluster, "pulValue"=→"pulValue":u32)  [unwired: 5 in, 2 out]
        n45 = call <vilib>:"Clear Errors.vi"("error in (no error)"=w99) -> ("error out"=w102:errorcluster)  [unwired: 5 in, 1 out]
        n46 = control-ref of="Get Com Param"() -> (w105:refnum<vi>)
        n47 = property class="Bool (strict)"(reference=w105, error in=w102, "Value"=FALSE) -> (error out=w103:errorcluster)  [unwired: 1 out]
        n48 = Merge Errors(w99, w103) -> (w104:errorcluster)
      }
      frame "Set Frame Param" {
        n49 = call "BISS Set Frame Param.vi"("ulValue"="ulValue", "Error In"=w113, "ulParam"="BISS_FrameParamEnum", "ulDataChannel"="ulDataChannel", "ulBISSHandle"=w112) -> ("Error Out"=w108:errorcluster)  [unwired: 4 in, 2 out]
        n50 = call <vilib>:"Clear Errors.vi"("error in (no error)"=w108) -> ("error out"=w114:errorcluster)  [unwired: 5 in, 1 out]
        n51 = control-ref of="Set Frame Param"() -> (w117:refnum<vi>)
        n52 = property class="Bool (strict)"(reference=w117, error in=w114, "Value"=FALSE) -> (error out=w115:errorcluster)  [unwired: 1 out]
        n53 = Merge Errors(w108, w115) -> (w116:errorcluster)
      }
      frame "Get Frame Param" {
        n54 = call "BISS Get Frame Param.vi"("Error In"=w125, "ulParam"="BISS_FrameParamEnum", "ulDataChannel"="ulDataChannel", "ulBISSHandle"=w124) -> ("Error Out"=w120:errorcluster, "pulValue"=→"pulValue":u32)  [unwired: 4 in, 2 out]
        n55 = call <vilib>:"Clear Errors.vi"("error in (no error)"=w120) -> ("error out"=w126:errorcluster)  [unwired: 5 in, 1 out]
        n56 = control-ref of="Get Frame Param"() -> (w129:refnum<vi>)
        n57 = property class="Bool (strict)"(reference=w129, error in=w126, "Value"=FALSE) -> (error out=w127:errorcluster)  [unwired: 1 out]
        n58 = Merge Errors(w120, w127) -> (w128:errorcluster)
      }
      frame "Write Master Params" {
        n59 = call "BISS Write Master Params.vi"("Error In"=w135, "ulBISSHandle"=w133) -> ("Error Out"=w134:errorcluster)  [unwired: 7 in, 2 out]
        n60 = call <vilib>:"Clear Errors.vi"("error in (no error)"=w134) -> ("error out"=w136:errorcluster)  [unwired: 5 in, 1 out]
        n61 = control-ref of="Write Master Params"() -> (w132:refnum<vi>)
        n62 = property class="Bool (strict)"(reference=w132, error in=w136, "Value"=FALSE) -> (error out=w137:errorcluster)  [unwired: 1 out]
        n63 = Merge Errors(w134, w137) -> (w138:errorcluster)
      }
      frame "Set FTDI Freq" {
        n64 = call "BISS Set Ftdi Freq.vi"("Error In"=w146, "ulFreqL"="ulFreqL", "ulFreqH"="ulFreqH", "ulBISSHandle"=w144) -> ("Error Out"=w145:errorcluster)  [unwired: 6 in, 1 out]
        n65 = call <vilib>:"Clear Errors.vi"("error in (no error)"=w145) -> ("error out"=w150:errorcluster)  [unwired: 5 in, 1 out]
        n66 = control-ref of="Set FTDI Freq"() -> (w141:refnum<vi>)
        n67 = property class="Bool (strict)"(reference=w141, error in=w150, "Value"=FALSE) -> (error out=w148:errorcluster)  [unwired: 1 out]
        n68 = Merge Errors(w145, w148) -> (w147:errorcluster)
      }
      frame "Init BiSS Comm" {
        n69 = call "BISS Init Biss Comm.vi"("Error In"=w156, "ulBiSSHandle"=w155) -> ("Error Out"=w154:errorcluster)  [unwired: 7 in, 2 out]
        n70 = call <vilib>:"Clear Errors.vi"("error in (no error)"=w154) -> ("error out"=w157:errorcluster)  [unwired: 5 in, 1 out]
        n71 = control-ref of="Init BiSS Comm"() -> (w158:refnum<vi>)
        n72 = property class="Bool (strict)"(reference=w158, error in=w157, "Value"=FALSE) -> (error out=w153:errorcluster)  [unwired: 1 out]
        n73 = Merge Errors(w154, w153) -> (w152:errorcluster)
      }
      frame "Write Slave Register" {
        n74 = call "BISS Write Slave Register.vi"("pulRegisterContent"="pulRegisterContent", "pulNumberOfBytes"="pulNumberOfBytes", "ulRegisterAddress"="ulRegisterAddress", "Error In"=w169, "ulSlaveId"="ulSlaveId", "ulProtocol"="ulProtocol", "ulBISSHandle"=w167) -> ("Error Out"=w168:errorcluster, "pulNumberOfBytes out"=w161:u32)  [unwired: 1 in, 2 out]
        n75 = property on="pulNumberOfBytes" class="DigNum (strict)"("Value"=w161) -> ()  [unwired: 2 in, 2 out]
        n76 = call <vilib>:"Clear Errors.vi"("error in (no error)"=w168) -> ("error out"=w172:errorcluster)  [unwired: 5 in, 1 out]
        n77 = control-ref of="Write Slave Register"() -> (w173:refnum<vi>)
        n78 = property class="Bool (strict)"(reference=w173, error in=w172, "Value"=FALSE) -> (error out=w171:errorcluster)  [unwired: 1 out]
        n79 = Merge Errors(w168, w171) -> (w170:errorcluster)
      }
      frame "Read Slave Register" {
        n80 = call "BISS Read Slave Register.vi"("pulNumberOfBytes"="pulNumberOfBytes", "ulRegisterAddress"="ulRegisterAddress", "Error In"=w184, "ulSlaveId"="ulSlaveId", "ulProtocol"="ulProtocol", "ulBISSHandle"=w185) -> ("Error Out"=w183:errorcluster, "pulRegisterContent"=→"pulRegisterContent":u32[], "pulNumberOfBytes"=w177:u32)  [unwired: 1 in, 2 out]
        n81 = property on="pulNumberOfBytes" class="DigNum (strict)"("Value"=w177) -> ()  [unwired: 2 in, 2 out]
        n82 = call <vilib>:"Clear Errors.vi"("error in (no error)"=w183) -> ("error out"=w187:errorcluster)  [unwired: 5 in, 1 out]
        n83 = control-ref of="Read Slave Register"() -> (w188:refnum<vi>)
        n84 = property class="Bool (strict)"(reference=w188, error in=w187, "Value"=FALSE) -> (error out=w186:errorcluster)  [unwired: 1 out]
        n85 = Merge Errors(w183, w186) -> (w182:errorcluster)
      }
      frame "Read SCD" {
        n86 = call "BISS Read SCD.vi"("Error In"=w198, "ulStartControlFrame"="ulStartControlFrame", "ulBISSHandle"=w196) -> ("Error Out"=w197:errorcluster, "pulDataScdL"=→"pulDataScdL":u32[], "pulDataScdH"=→"pulDataScdH":u32[], "pulScdValid"=→"pulScdValid":u32, "pulControlFrameEnd"=→"pulControlFrameEnd":u32)  [unwired: 3 in, 1 out]
        n87 = call <vilib>:"Clear Errors.vi"("error in (no error)"=w197) -> ("error out"=w201:errorcluster)  [unwired: 5 in, 1 out]
        n88 = control-ref of="Read SCD"() -> (w202:refnum<vi>)
        n89 = property class="Bool (strict)"(reference=w202, error in=w201, "Value"=FALSE) -> (error out=w199:errorcluster)  [unwired: 1 out]
        n90 = Merge Errors(w197, w199) -> (w200:errorcluster)
      }
      frame "Send Command" {
        n91 = call "BISS Send Command.vi"("Error In"=w208, "ulCmd"="ulCmd", "ulIds"="ulIds", "ulBISSHandle"=w209) -> ("Error Out"=w207:errorcluster)  [unwired: 5 in, 2 out]
        n92 = call <vilib>:"Clear Errors.vi"("error in (no error)"=w207) -> ("error out"=w212:errorcluster)  [unwired: 5 in, 1 out]
        n93 = control-ref of="Send Command"() -> (w213:refnum<vi>)
        n94 = property class="Bool (strict)"(reference=w213, error in=w212, "Value"=FALSE) -> (error out=w211:errorcluster)  [unwired: 1 out]
        n95 = Merge Errors(w207, w211) -> (w210:errorcluster)
      }
      frame "Set Slave Label" {
        n96 = call "BISS Set Slave Label.vi"("pcManufacturerLabel"="pcManufacturerLabel", "pcCompleteLabel"="pcCompleteLabel", "Error In"=w222, "pcSlaveLabel"="pcSlaveLabel", "ulSlave"="ulSlave", "ulBISSHandle"=w221) -> ("Error Out"=w220:errorcluster)  [unwired: 4 in, 1 out]
        n97 = call <vilib>:"Clear Errors.vi"("error in (no error)"=w220) -> ("error out"=w225:errorcluster)  [unwired: 5 in, 1 out]
        n98 = control-ref of="Set Slave Label"() -> (w226:refnum<vi>)
        n99 = property class="Bool (strict)"(reference=w226, error in=w225, "Value"=FALSE) -> (error out=w223:errorcluster)  [unwired: 1 out]
        n100 = Merge Errors(w220, w223) -> (w224:errorcluster)
      }
      frame "Get Slave Label" {
        n101 = call "BISS Get Slave Label.vi"("Error In"=w235, "ulSlave"="ulSlave 2", "ulBISSHandle"=w236) -> ("Error Out"=w234:errorcluster, "pcSlaveLabel"=→"pcSlaveLabel 2":string, "pcManufacturerLabel"=→"pcManufacturerLabel 2":string, "pcCompleteLabel"=→"pcCompleteLabel 2":string)  [unwired: 3 in, 2 out]
        n102 = call <vilib>:"Clear Errors.vi"("error in (no error)"=w234) -> ("error out"=w237:errorcluster)  [unwired: 5 in, 1 out]
        n103 = control-ref of="Get Slave Label"() -> (w233:refnum<vi>)
        n104 = property class="Bool (strict)"(reference=w233, error in=w237, "Value"=FALSE) -> (error out=w238:errorcluster)  [unwired: 1 out]
        n105 = Merge Errors(w234, w238) -> (w239:errorcluster)
      }
      frame "Set SCD Content Labels" {
        n106 = call "BISS Set SCD Content Labels.vi"("pcScdContentUnit"="pcScdContentUnit", "pcScdContentLabel"="pcScdContentLabel", "Error In"=w248, "ulContentIndex"="ulContentIndex", "ulDataChannel"="ulDataChannel", "ulBISSHandle"=w246) -> ("Error Out"=w247:errorcluster)  [unwired: 3 in, 2 out]
        n107 = call <vilib>:"Clear Errors.vi"("error in (no error)"=w247) -> ("error out"=w251:errorcluster)  [unwired: 5 in, 1 out]
        n108 = control-ref of="Set SCD Content Labels"() -> (w252:refnum<vi>)
        n109 = property class="Bool (strict)"(reference=w252, error in=w251, "Value"=FALSE) -> (error out=w249:errorcluster)  [unwired: 1 out]
        n110 = Merge Errors(w247, w249) -> (w250:errorcluster)
      }
      frame "Get SCD Content Labels" {
        n111 = call "BISS Get SCD Content Labels.vi"("Error In"=w261, "ulContentIndex"="ulContentIndex", "ulDataChannel"="ulDataChannel", "ulBISSHandle"=w259) -> ("Error Out"=w260:errorcluster, "pcSCDContentUnit"=→"pcSCDContentUnit":string, "pcSCDContentLabel"=→"pcSCDContentLabel":string)  [unwired: 3 in, 2 out]
        n112 = call <vilib>:"Clear Errors.vi"("error in (no error)"=w260) -> ("error out"=w264:errorcluster)  [unwired: 5 in, 1 out]
        n113 = control-ref of="Get SCD Content Labels"() -> (w265:refnum<vi>)
        n114 = property class="Bool (strict)"(reference=w265, error in=w264, "Value"=FALSE) -> (error out=w262:errorcluster)  [unwired: 1 out]
        n115 = Merge Errors(w260, w262) -> (w263:errorcluster)
      }
      frame "Get SCD Content" {
        n116 = call "BISS Get SCD Content.vi"("Error In"=w272, "ulDataChannel"="ulDataChannel", "ulBISSHandle"=w270) -> ("Error Out"=w271:errorcluster, "pulScdContentValues"=→"pulScdContentValues":u32[])  [unwired: 5 in, 2 out]
        n117 = call <vilib>:"Clear Errors.vi"("error in (no error)"=w271) -> ("error out"=w275:errorcluster)  [unwired: 5 in, 1 out]
        n118 = control-ref of="Get SCD Content"() -> (w276:refnum<vi>)
        n119 = property class="Bool (strict)"(reference=w276, error in=w275, "Value"=FALSE) -> (error out=w273:errorcluster)  [unwired: 1 out]
        n120 = Merge Errors(w271, w273) -> (w274:errorcluster)
      }
      frame "Get SCD Content Ex" {
        n121 = call "BISS Get SCD Content Ex.vi"("Error In"=w283, "ulDataChannel"="ulDataChannel", "ulBISSHandle"=w281) -> ("Error Out"=w282:errorcluster, "pulScdContentValues"=→"pulScdContentValues":u64[])  [unwired: 6 in, 1 out]
        n122 = call <vilib>:"Clear Errors.vi"("error in (no error)"=w282) -> ("error out"=w286:errorcluster)  [unwired: 5 in, 1 out]
        n123 = control-ref of="Get SCD Content Ex"() -> (w287:refnum<vi>)
        n124 = property class="Bool (strict)"(reference=w287, error in=w286, "Value"=FALSE) -> (error out=w284:errorcluster)  [unwired: 1 out]
        n125 = Merge Errors(w282, w284) -> (w285:errorcluster)
      }
      frame "Set SCD Content Params" {
        n126 = call "BISS Set SCD Content Params.vi"("pScdContentItems"="pScdContentItems", "Error In"=w295, "ulContentIndex"="ulContentIndex", "ulDataChannel"="ulDataChannel", "ulBISSHandle"=w293) -> ("Error Out"=w294:errorcluster)  [unwired: 4 in, 2 out]
        n127 = call <vilib>:"Clear Errors.vi"("error in (no error)"=w294) -> ("error out"=w298:errorcluster)  [unwired: 5 in, 1 out]
        n128 = control-ref of="Set SCD Content Params"() -> (w299:refnum<vi>)
        n129 = property class="Bool (strict)"(reference=w299, error in=w298, "Value"=FALSE) -> (error out=w296:errorcluster)  [unwired: 1 out]
        n130 = Merge Errors(w294, w296) -> (w297:errorcluster)
      }
      frame "Get SCD Content Params" {
        n131 = call "BISS Get SCD Content Params.vi"("Error In"=w307, "ulContentIndex"="ulContentIndex", "ulDataChannel"="ulDataChannel", "ulBISSHandle"=w305) -> ("Error Out"=w306:errorcluster, "pScdContentItems out"=→"pScdContentItems":T7)  [unwired: 4 in, 2 out]
        n132 = call <vilib>:"Clear Errors.vi"("error in (no error)"=w306) -> ("error out"=w310:errorcluster)  [unwired: 5 in, 1 out]
        n133 = control-ref of="Get SCD Content Params"() -> (w311:refnum<vi>)
        n134 = property class="Bool (strict)"(reference=w311, error in=w310, "Value"=FALSE) -> (error out=w308:errorcluster)  [unwired: 1 out]
        n135 = Merge Errors(w306, w308) -> (w309:errorcluster)
      }
      frame "Read SCD Frames" {
        n136 = Tick Count (ms)() -> (millisecond timer value=w317:u32)
        n137 = call "Tovey9150_OpenPort.vi"() -> ("error out"=w315:errorcluster, "Serial Port"=w316:refnum<visa-resource-name>)  [unwired: 1 in, 9 out]
        n138 = while {
          tunnel: w319 -> [w362]
          shift-right: [w361] -> w318
          shift-left: w320 -> [w363]
          tunnel: [w340] -> _
          tunnel: w317 -> [w339]
          tunnel: w316 -> [w329]
          tunnel: w315 -> [w328]
          tunnel: [w324] -> w314
          stop <- "stop" stop-if-true
          n139 = call "Tovey9150_GetValues.vi"("error in (no error)"=w328, "Send"="@001V5006061", "Read Serial Port"=w329) -> ("error out"=→"error out":errorcluster, "Rcv"=w333:string, "Serial Port"=w324:refnum<visa-resource-name>)  [unwired: 6 out]
          "Load Cells Display" <- w333
          n140 = Tick Count (ms)() -> (millisecond timer value=w340:u32)
          n141 = call "BISS Read SCD Frames.vi"("Error In"=w363, "ulCycleCnt"="ulCycleCnt", "ulBISSHandle"=w362) -> ("Error Out"=w353:errorcluster, "pulDataScdL"=w358:u32[], "pulDataScdH"=→"pulDataScdH":u32[], "pulTimestamp"=→"pulTimestamp":u32[], "pulStatus"=→"pulStatus":u32[])  [unwired: 3 in, 1 out]
          n142 = Subtract(x=w340, y=w339) -> (x-y=→"Loop Time [ms]":u32)
          n143 = Wait Until Next ms Multiple(millisecond multiple="Update Time [ms]") -> ()  [unwired: 1 out]
          n144 = Scan From String(format string="@ 001 LoadA %f kN LoadB %f kN " ("Rcv"), input string=w333) -> (output 1=w330:dbl, output 2=→"Load B [kN]":dbl)  [unwired: 2 in, 5 out]
          "Load A [kN]" <- w330
          n145 = Logical Shift(y=-2, x=w358) -> (x << y=w359:u32[])
          n146 = To Single Precision Float(number=w359) -> (single precision float=w360:sgl[])
          n147 = Build Array(w330) -> (w322:dbl[])
          n148 = Get Date/Time In Seconds() -> (seconds since 1Jan1904=w345:timestamp)
          n149 = Get Date/Time In Seconds() -> (seconds since 1Jan1904=w326:timestamp)
          n150 = call <vilib>:"Clear Errors.vi"("error in (no error)"=w353) -> ("error out"=w351:errorcluster)  [unwired: 5 in, 1 out]
          n151 = Divide(x=w360, y=1000000) -> (x/y=w323:sgl[])
          "pulDataScdL" <- w323
          n152 = Bundle By Name("t0"=w345, "Y"=w323, "dt"=1) -> (→"Displacement vs Time":waveform(sgl))  [unwired: 1 in]
          n153 = control-ref of="Read SCD Frames"() -> (w350:refnum<vi>)
          n154 = Bundle By Name("t0"=w326, "Y"=w322, "dt"=1) -> (→"Load A vs Time":waveform(dbl))  [unwired: 1 in]
          n155 = Build Array(w323) -> ()  [unwired: 1 out]
          n156 = property class="Bool (strict)"(reference=w350, error in=w351, "Value"=FALSE) -> (error out=w352:errorcluster)  [unwired: 1 out]
          n157 = Merge Errors(w353, w352) -> (w361:errorcluster)
          n158 = call "Convert to Dynamic Data"("Array"="data") -> ("Dynamic Data Type"=w337:dynamicdata)  [unwired: 3 out]
          n159 = call "DAQNavi Assistant"("data in(DDT)"=w337) -> ("error out"=→"error out 2":errorcluster)  [unwired: 2 in, 16 out]
        }
        n160 = VISA Close(VISA resource name=w314) -> ()  [unwired: 1 in, 1 out]
      }
      frame "Get SCD Frame" {
        n161 = call "BiSS Get SCD Frame.vi"("Error In"=w370, "ulFrameIndex"="ulFrameIndex", "ulBISSHandle"=w371) -> ("Error Out"=w369:errorcluster, "pulDataScdL"=→"pulDataScdL":u32[], "pulDataScdH"=→"pulDataScdH":u32[], "pulStatus"=→"pulStatus":u32, "pulTimestamp"=→"pulTimestamp":u32)  [unwired: 2 in, 2 out]
        n162 = call <vilib>:"Clear Errors.vi"("error in (no error)"=w369) -> ("error out"=w374:errorcluster)  [unwired: 5 in, 1 out]
        n163 = control-ref of="Get SCD Frame"() -> (w375:refnum<vi>)
        n164 = property class="Bool (strict)"(reference=w375, error in=w374, "Value"=FALSE) -> (error out=w372:errorcluster)  [unwired: 1 out]
        n165 = Merge Errors(w369, w372) -> (w373:errorcluster)
      }
      frame "Get SCD Frame Ex" {
        n166 = call "BISS Get SCD Frame Ex.vi"("ulCycleCount"="ulCycleCount", "Error In"=w386, "ulDataChannel"="ulDataChannel", "ulBISSHandle"=w384) -> ("Error Out"=w385:errorcluster, "pulDataScdL"=→"pulDataScdL":u32[], "pulDataScdH"=→"pulDataScdH":u32[], "pulTimestamp"=→"pulTimestamp":u32[], "pulStatus"=→"pulStatus":u32[])  [unwired: 2 in, 1 out]
        n167 = call <vilib>:"Clear Errors.vi"("error in (no error)"=w385) -> ("error out"=w389:errorcluster)  [unwired: 5 in, 1 out]
        n168 = control-ref of="Get SCD Frame Ex"() -> (w390:refnum<vi>)
        n169 = property class="Bool (strict)"(reference=w390, error in=w389, "Value"=FALSE) -> (error out=w387:errorcluster)  [unwired: 1 out]
        n170 = Merge Errors(w385, w387) -> (w388:errorcluster)
      }
      frame "Get SCD Frame Content" {
        n171 = call "BISS Get SCD Frame Content.vi"("ulCycleCount"="ulCycleCount", "Error In"=w399, "ulContentIndex"="ulContentIndex", "ulDataChannel"="ulDataChannel", "ulBISSHandle"=w397) -> ("Error Out"=w398:errorcluster, "pulValues"=→"pulValues":u32[])  [unwired: 3 in, 2 out]
        n172 = call <vilib>:"Clear Errors.vi"("error in (no error)"=w398) -> ("error out"=w402:errorcluster)  [unwired: 5 in, 1 out]
        n173 = control-ref of="Get SCD Frame Content"() -> (w403:refnum<vi>)
        n174 = property class="Bool (strict)"(reference=w403, error in=w402, "Value"=FALSE) -> (error out=w400:errorcluster)  [unwired: 1 out]
        n175 = Merge Errors(w398, w400) -> (w401:errorcluster)
      }
      frame "Get SCD Frame Content Ex" {
        n176 = call "BISS Get SCD Frame Content Ex.vi"("ulCycleCount"="ulCycleCount", "Error In"=w417, "ulContentIndex"="ulContentIndex", "ulDataChannel"="ulDataChannel", "ulBISSHandle"=w416) -> ("Error Out"=w408:errorcluster, "pulValues"=→"pulValues":u64[])  [unwired: 4 in, 1 out]
        n177 = call <vilib>:"Clear Errors.vi"("error in (no error)"=w408) -> ("error out"=w411:errorcluster)  [unwired: 5 in, 1 out]
        n178 = control-ref of="Get SCD Frame Content Ex"() -> (w406:refnum<vi>)
        n179 = property class="Bool (strict)"(reference=w406, error in=w411, "Value"=FALSE) -> (error out=w410:errorcluster)  [unwired: 1 out]
        n180 = Merge Errors(w408, w410) -> (w407:errorcluster)
      }
      frame "Set EDS Param" {
        n181 = call "BISS Set EDS Param.vi"("Error In"=w423, "ulValue"="ulValue", "ulParam"="BISS_EdsParamEnum", "ulBISSHandle"=w421) -> ("Error Out"=w422:errorcluster)  [unwired: 6 in, 1 out]
        n182 = call <vilib>:"Clear Errors.vi"("error in (no error)"=w422) -> ("error out"=w426:errorcluster)  [unwired: 5 in, 1 out]
        n183 = control-ref of="Set EDS Param"() -> (w427:refnum<vi>)
        n184 = property class="Bool (strict)"(reference=w427, error in=w426, "Value"=FALSE) -> (error out=w425:errorcluster)  [unwired: 1 out]
        n185 = Merge Errors(w422, w425) -> (w424:errorcluster)
      }
      frame "Get EDS Param" {
        n186 = call "BISS Get EDS Param.vi"("Error In"=w434, "ulParam"="BISS_EdsParamEnum", "ulBISSHandle"=w432) -> ("Error Out"=w433:errorcluster, "pulValue"=→"pulValue":u32)  [unwired: 6 in, 1 out]
        n187 = call <vilib>:"Clear Errors.vi"("error in (no error)"=w433) -> ("error out"=w437:errorcluster)  [unwired: 5 in, 1 out]
        n188 = control-ref of="Get EDS Param"() -> (w438:refnum<vi>)
        n189 = property class="Bool (strict)"(reference=w438, error in=w437, "Value"=FALSE) -> (error out=w436:errorcluster)  [unwired: 1 out]
        n190 = Merge Errors(w433, w436) -> (w435:errorcluster)
      }
      frame "Set EDS Register" {
        n191 = call "BISS Set EDS Register.vi"("Error In"=w444, "ulValue"="ulValue", "ulAdr"="ulAdr", "ulBISSHandle"=w445) -> ("Error Out"=w443:errorcluster)  [unwired: 6 in, 1 out]
        n192 = call <vilib>:"Clear Errors.vi"("error in (no error)"=w443) -> ("error out"=w448:errorcluster)  [unwired: 5 in, 1 out]
        n193 = control-ref of="Set EDS Register"() -> (w449:refnum<vi>)
        n194 = property class="Bool (strict)"(reference=w449, error in=w448, "Value"=FALSE) -> (error out=w447:errorcluster)  [unwired: 1 out]
        n195 = Merge Errors(w443, w447) -> (w446:errorcluster)
      }
      frame "Get EDS Register" {
        n196 = call "BISS Get EDS Register.vi"("Error In"=w455, "ulAdr"="ulAdr", "ulBISSHandle"=w456) -> ("Error Out"=w454:errorcluster, "pulValue"=→"pulValue":u32)  [unwired: 6 in, 1 out]
        n197 = call <vilib>:"Clear Errors.vi"("error in (no error)"=w454) -> ("error out"=w459:errorcluster)  [unwired: 5 in, 1 out]
        n198 = control-ref of="Get EDS Register"() -> (w460:refnum<vi>)
        n199 = property class="Bool (strict)"(reference=w460, error in=w459, "Value"=FALSE) -> (error out=w458:errorcluster)  [unwired: 1 out]
        n200 = Merge Errors(w454, w458) -> (w457:errorcluster)
      }
      frame "Read EDS Params" {
        n201 = call "BISS Read EDS Params.vi"("Error In"=w466, "ulSlaveId"="ulSlaveId", "ulBISSHandle"=w464) -> ("Error Out"=w465:errorcluster)  [unwired: 7 in, 1 out]
        n202 = call <vilib>:"Clear Errors.vi"("error in (no error)"=w465) -> ("error out"=w469:errorcluster)  [unwired: 5 in, 1 out]
        n203 = control-ref of="Read EDS Params"() -> (w470:refnum<vi>)
        n204 = property class="Bool (strict)"(reference=w470, error in=w469, "Value"=FALSE) -> (error out=w468:errorcluster)  [unwired: 1 out]
        n205 = Merge Errors(w465, w468) -> (w467:errorcluster)
      }
      frame "Write EDS Params" {
        n206 = call "BISS Write EDS Params.vi"("Error In"=w476, "ulSlaveId"="ulSlaveId", "ulBISSHandle"=w474) -> ("Error Out"=w475:errorcluster)  [unwired: 7 in, 1 out]
        n207 = call <vilib>:"Clear Errors.vi"("error in (no error)"=w475) -> ("error out"=w479:errorcluster)  [unwired: 5 in, 1 out]
        n208 = control-ref of="Write EDS Params"() -> (w480:refnum<vi>)
        n209 = property class="Bool (strict)"(reference=w480, error in=w479, "Value"=FALSE) -> (error out=w478:errorcluster)  [unwired: 1 out]
        n210 = Merge Errors(w475, w478) -> (w477:errorcluster)
      }
      frame "Get DLL Version" {
        n211 = call "BISS Get DLL Version.vi"("Error In"=w485) -> ("Error Out"=w484:errorcluster, "pulDllVersion"=→"pulDllVersion":u32[])  [unwired: 7 in, 2 out]
        n212 = call <vilib>:"Clear Errors.vi"("error in (no error)"=w484) -> ("error out"=w489:errorcluster)  [unwired: 5 in, 1 out]
        n213 = control-ref of="Get DLL Version"() -> (w490:refnum<vi>)
        n214 = property class="Bool (strict)"(reference=w490, error in=w489, "Value"=FALSE) -> (error out=w488:errorcluster)  [unwired: 1 out]
        n215 = Merge Errors(w484, w488) -> (w487:errorcluster)
      }
      frame "Calculate CRC" {
        n216 = call "BISS Calculate CRC.vi"("ulByteCount"="ulByteCount", "Error In"=w499, "pulData"="pulData", "ulCrcPoly"="ulCrcPoly", "ulBISSHandle"=w497) -> ("Error Out"=w498:errorcluster, "pulCheckSum"=→"pulCheckSum":u32)  [unwired: 4 in, 1 out]
        n217 = call <vilib>:"Clear Errors.vi"("error in (no error)"=w498) -> ("error out"=w502:errorcluster)  [unwired: 5 in, 1 out]
        n218 = control-ref of="Calculate CRC"() -> (w503:refnum<vi>)
        n219 = property class="Bool (strict)"(reference=w503, error in=w502, "Value"=FALSE) -> (error out=w501:errorcluster)  [unwired: 1 out]
        n220 = Merge Errors(w498, w501) -> (w500:errorcluster)
      }
      frame "Calculate CRC Ex" {
        n221 = call "BISS Calculate CRC Ex.vi"("ulCRCStartValue"="ulCRCStartValue", "ulByteCount"="ulByteCount", "Error In"=w513, "pulData"="pulData", "ulCrcPoly"="ulCrcPoly", "ulBISSHandle"=w511) -> ("Error Out"=w512:errorcluster, "pulCheckSum"=→"pulCheckSum":u32)  [unwired: 3 in, 1 out]
        n222 = call <vilib>:"Clear Errors.vi"("error in (no error)"=w512) -> ("error out"=w516:errorcluster)  [unwired: 5 in, 1 out]
        n223 = control-ref of="Calculate CRC Ex"() -> (w517:refnum<vi>)
        n224 = property class="Bool (strict)"(reference=w517, error in=w516, "Value"=FALSE) -> (error out=w515:errorcluster)  [unwired: 1 out]
        n225 = Merge Errors(w512, w515) -> (w514:errorcluster)
      }
      frame "Save DLL Config" {
        n226 = Path To String(path="pcFilename") -> (string=w522:string)
        n227 = call "BISS Save DLL Config.vi"("Error In"=w524, "pcCfgFilename"=w522, "ulBISSHandle"=w525) -> ("Error Out"=w523:errorcluster)  [unwired: 7 in, 1 out]
        n228 = call <vilib>:"Clear Errors.vi"("error in (no error)"=w523) -> ("error out"=w528:errorcluster)  [unwired: 5 in, 1 out]
        n229 = control-ref of="Save DLL Config"() -> (w520:refnum<vi>)
        n230 = property class="Bool (strict)"(reference=w520, error in=w528, "Value"=FALSE) -> (error out=w527:errorcluster)  [unwired: 1 out]
        n231 = Merge Errors(w523, w527) -> (w526:errorcluster)
      }
      frame "Load DLL Config" {
        n232 = Path To String(path="pcFilename 2") -> (string=w533:string)
        n233 = call "BISS Load DLL Config.vi"("Error In"=w535, "pcCfgFilename"=w533, "ulBISSHandle"=w536) -> ("Error Out"=w534:errorcluster)  [unwired: 7 in, 1 out]
        n234 = call <vilib>:"Clear Errors.vi"("error in (no error)"=w534) -> ("error out"=w539:errorcluster)  [unwired: 5 in, 1 out]
        n235 = control-ref of="Load DLL Config"() -> (w532:refnum<vi>)
        n236 = property class="Bool (strict)"(reference=w532, error in=w539, "Value"=FALSE) -> (error out=w538:errorcluster)  [unwired: 1 out]
        n237 = Merge Errors(w534, w538) -> (w537:errorcluster)
      }
      frame "Get Last Error" {
        n238 = call "BISS Get Last Error.vi"("Error In"=w547, "ulBISSHandle"=w545) -> ("Error Out"=w546:errorcluster, "pulErrorType"=→"BISS_ErrorTypeEnum":u32, "pulLastError"=→"pulLastError":u32, "pcErrorText"=→"pcErrorText":string)  [unwired: 5 in, 1 out]
        n239 = call <vilib>:"Clear Errors.vi"("error in (no error)"=w546) -> ("error out"=w550:errorcluster)  [unwired: 5 in, 1 out]
        n240 = control-ref of="Get Last Error"() -> (w551:refnum<vi>)
        n241 = property class="Bool (strict)"(reference=w551, error in=w550, "Value"=FALSE) -> (error out=w549:errorcluster)  [unwired: 1 out]
        n242 = Merge Errors(w546, w549) -> (w548:errorcluster)
      }
      frame "Get MB3U Pins" {
        n243 = call "BISS Get MB3U Pins.vi"("Error In"=w558, "ulBISSHandle"=w556) -> ("Error Out"=w557:errorcluster, "pulValue"=→"pulValue":u32, "pulDir"=→"pulDir":u32)  [unwired: 6 in, 1 out]
        n244 = call <vilib>:"Clear Errors.vi"("error in (no error)"=w557) -> ("error out"=w561:errorcluster)  [unwired: 5 in, 1 out]
        n245 = control-ref of="Get MB3U Pins"() -> (w562:refnum<vi>)
        n246 = property class="Bool (strict)"(reference=w562, error in=w561, "Value"=FALSE) -> (error out=w560:errorcluster)  [unwired: 1 out]
        n247 = Merge Errors(w557, w560) -> (w559:errorcluster)
      }
      frame "Set MB3U Pins" {
        n248 = call "BISS Set MB3U Pins.vi"("Error In"=w569, "ulValue"="ulValue", "ulDir"="ulDir", "ulBISSHandle"=w567) -> ("Error Out"=w568:errorcluster)  [unwired: 6 in, 1 out]
        n249 = call <vilib>:"Clear Errors.vi"("error in (no error)"=w568) -> ("error out"=w572:errorcluster)  [unwired: 5 in, 1 out]
        n250 = control-ref of="Set MB3U Pins"() -> (w573:refnum<vi>)
        n251 = property class="Bool (strict)"(reference=w573, error in=w572, "Value"=FALSE) -> (error out=w571:errorcluster)  [unwired: 1 out]
        n252 = Merge Errors(w568, w571) -> (w570:errorcluster)
      }
      frame "Write Master Register" {
        n253 = call "BISS Write Master Register.vi"("Error In"=w580, "ulRegisterContent"="ulRegisterContent", "ulRegisterAddress"="ulRegisterAddress", "ulBISSHandle"=w578) -> ("Error Out"=w579:errorcluster)  [unwired: 5 in, 2 out]
        n254 = call <vilib>:"Clear Errors.vi"("error in (no error)"=w579) -> ("error out"=w583:errorcluster)  [unwired: 5 in, 1 out]
        n255 = control-ref of="Write Master Register"() -> (w584:refnum<vi>)
        n256 = property class="Bool (strict)"(reference=w584, error in=w583, "Value"=FALSE) -> (error out=w582:errorcluster)  [unwired: 1 out]
        n257 = Merge Errors(w579, w582) -> (w581:errorcluster)
      }
      frame "Read Master Register" {
        n258 = call "BISS Read Master Register.vi"("Error In"=w591, "ulRegisterAddress"="ulRegisterAddress", "ulBISSHandle"=w589) -> ("Error Out"=w590:errorcluster, "pulRegisterContent"=→"pulRegisterContent":u32)  [unwired: 5 in, 2 out]
        n259 = call <vilib>:"Clear Errors.vi"("error in (no error)"=w590) -> ("error out"=w594:errorcluster)  [unwired: 5 in, 1 out]
        n260 = control-ref of="Read Master Register"() -> (w595:refnum<vi>)
        n261 = property class="Bool (strict)"(reference=w595, error in=w594, "Value"=FALSE) -> (error out=w593:errorcluster)  [unwired: 1 out]
        n262 = Merge Errors(w590, w593) -> (w592:errorcluster)
      }
      frame "Get Master Register" {
        n263 = call "BISS Get Master Register.vi"("Error In"=w602, "ulRegisterAddress"="ulRegisterAddress", "ulBISSHandle"=w600) -> ("Error Out"=w601:errorcluster, "pulRegisterContent"=→"pulRegisterContent":u32)  [unwired: 5 in, 2 out]
        n264 = call <vilib>:"Clear Errors.vi"("error in (no error)"=w601) -> ("error out"=w605:errorcluster)  [unwired: 5 in, 1 out]
        n265 = control-ref of="Get Master Register"() -> (w606:refnum<vi>)
        n266 = property class="Bool (strict)"(reference=w606, error in=w605, "Value"=FALSE) -> (error out=w604:errorcluster)  [unwired: 1 out]
        n267 = Merge Errors(w601, w604) -> (w603:errorcluster)
      }
      frame "Save Master Config" {
        n268 = Path To String(path="pcFilename") -> (string=w609:string)
        n269 = call "BISS Save Master Config.vi"("Error In"=w613, "pcCfgFilename"=w609, "ulBISSHandle"=w611) -> ("Error Out"=w612:errorcluster)  [unwired: 7 in, 1 out]
        n270 = call <vilib>:"Clear Errors.vi"("error in (no error)"=w612) -> ("error out"=w616:errorcluster)  [unwired: 5 in, 1 out]
        n271 = control-ref of="Save Master Config"() -> (w617:refnum<vi>)
        n272 = property class="Bool (strict)"(reference=w617, error in=w616, "Value"=FALSE) -> (error out=w615:errorcluster)  [unwired: 1 out]
        n273 = Merge Errors(w612, w615) -> (w614:errorcluster)
      }
      frame "Save Register" {
        n274 = Path To String(path="pcFilename") -> (string=w623:string)
        n275 = call "BISS Save Register.vi"("pulData"="pulData", "ulNumberOfBytes"="ulNumberOfBytes", "Error In"=w627, "ulStartAdr"="ulStartAdr", "pcFilename"=w623, "ulBISSHandle"=w625) -> ("Error Out"=w626:errorcluster)  [unwired: 4 in, 1 out]
        n276 = call <vilib>:"Clear Errors.vi"("error in (no error)"=w626) -> ("error out"=w630:errorcluster)  [unwired: 5 in, 1 out]
        n277 = control-ref of="Save Register"() -> (w631:refnum<vi>)
        n278 = property class="Bool (strict)"(reference=w631, error in=w630, "Value"=FALSE) -> (error out=w629:errorcluster)  [unwired: 1 out]
        n279 = Merge Errors(w626, w629) -> (w628:errorcluster)
      }
      frame "Load Register" {
        n280 = Path To String(path="pcFilename") -> (string=w637:string)
        n281 = call "BISS Load Register.vi"("ulNumberOfBytes"="ulNumberOfBytes", "Error In"=w641, "ulStartAdr"="ulStartAdr", "pcFilename"=w637, "ulBISSHandle"=w639) -> ("Error Out"=w640:errorcluster, "pulData"=→"pulData":u32[])  [unwired: 4 in, 1 out]
        n282 = call <vilib>:"Clear Errors.vi"("error in (no error)"=w640) -> ("error out"=w644:errorcluster)  [unwired: 5 in, 1 out]
        n283 = control-ref of="Load Register"() -> (w645:refnum<vi>)
        n284 = property class="Bool (strict)"(reference=w645, error in=w644, "Value"=FALSE) -> (error out=w643:errorcluster)  [unwired: 1 out]
        n285 = Merge Errors(w640, w643) -> (w642:errorcluster)
      }
      frame "Stop Demo" {
        n286 = Release Queue(queue=w654, error in (no error)=w655) -> (error out=w648:errorcluster)  [unwired: 1 in, 2 out]
        n287 = call <vilib>:"Clear Errors.vi"("error in (no error)"=w648) -> ("error out"=w651:errorcluster)  [unwired: 5 in, 1 out]
        n288 = control-ref of="Stop Button"() -> (w650:refnum<vi>)
        n289 = property class="Bool (strict)"(reference=w650, error in=w651, "Value"=FALSE) -> (error out=w652:errorcluster)  [unwired: 1 out]
        n290 = Merge Errors(w648, w652) -> (w653:errorcluster)
      }
    }
    n291 = call <vilib>:"Simple Error Handler.vi"("error in (no error)"=w13) -> ()  [unwired: 4 in, 5 out]
  }
  n292 = while {
    tunnel: w3 -> [w661]
    tunnel: w4 -> [w662]
    tunnel: FALSE -> [w659]
    stop <- w658 stop-if-true
    n293 = event shown="[18] \"Get Slave Label\": Value Change" {
      selector: _ -> [_ _ _ _ _ _ _ _ _ _ _ _ _ _ _ _ _ _ _ _ _ _ _ _ _ _ _ _ _ _ _ _ _ _ _ _ _ _ _ _ _ _ _ _ _ _ _ _ _ _ _]
      dyn-events: _ -> [_ _ _ _ _ _ _ _ _ _ _ _ _ _ _ _ _ _ _ _ _ _ _ _ _ _ _ _ _ _ _ _ _ _ _ _ _ _ _ _ _ _ _ _ _ _ _ _ _ _ _]
      timeout: _ -> [_ _ _ _ _ _ _ _ _ _ _ _ _ _ _ _ _ _ _ _ _ _ _ _ _ _ _ _ _ _ _ _ _ _ _ _ _ _ _ _ _ _ _ _ _ _ _ _ _ _ _]
      tunnel: w661 -> [w667 w672 w677 w682 w687 w691 w697 w702 w706 w712 w717 w722 w727 w732 w737 w742 w747 w752 w757 w762 w767 w772 w775 w780 w785 w790 w795 w800 w805 w811 w815 w820 w825 w830 w835 w840 w845 w850 w855 w860 w865 w870 w875 w880 w885 w890 w895 w900 w905 w910 w916]
      tunnel: [w666 w671 w676 w681 w686 w692 w696 w701 w707 w711 w716 w719 w726 w731 w736 w741 w746 w751 w756 w761 w766 w770 w773 w778 w783 w788 w793 w798 w803 w810 w813 w818 w823 w828 w833 w838 w843 w848 w853 w858 w863 w868 w873 w878 w883 w888 w893 w898 w903 w908 w914] -> w660
      tunnel: w662 -> [w665 w670 w675 w680 w685 w690 w695 w700 w705 w710 w715 w721 w725 w730 w735 w740 w745 w750 w755 w760 w765 w771 w774 w779 w784 w789 w794 w799 w804 w809 w814 w819 w824 w829 w834 w839 w844 w849 w854 w859 w864 w869 w874 w879 w884 w889 w894 w899 w904 w909 w915]
      tunnel: w659 -> [w663 w668 w673 w678 w683 w688 w693 w698 w703 w708 w713 w718 w723 w728 w733 w738 w743 w748 w753 w758 w763 w768 w777 w782 w787 w792 w797 w802 w807 w812 w817 w822 w827 w832 w837 w842 w847 w852 w857 w862 w867 w872 w877 w882 w887 w892 w897 w902 w907 w912 _]
      tunnel: [w663 w668 w673 w678 w683 w688 w693 w698 w703 w708 w713 w718 w723 w728 w733 w738 w743 w748 w753 w758 w763 w768 w777 w782 w787 w792 w797 w802 w807 w812 w817 w822 w827 w832 w837 w842 w847 w852 w857 w862 w867 w872 w877 w882 w887 w892 w897 w902 w907 w912 TRUE] -> w658
      event "Open": Value Change {
        n294 = event-data() -> ()  [unwired: 1 in, 1 out]
        n295 = Enqueue Element(queue=w665, element=BiSS_Interface_Demo_Functions."Open" ("Events"), error in (no error)=w667) -> (error out=w666:errorcluster)  [unwired: 1 in, 2 out]
      }
      event "Close": Value Change {
        n296 = event-data() -> ()  [unwired: 1 in, 1 out]
        n297 = Enqueue Element(queue=w670, element=BiSS_Interface_Demo_Functions."Close" ("Events"), error in (no error)=w672) -> (error out=w671:errorcluster)  [unwired: 1 in, 2 out]
      }
      event "Set Interface": Value Change {
        n298 = event-data() -> ()  [unwired: 1 in, 1 out]
        n299 = Enqueue Element(queue=w675, element=BiSS_Interface_Demo_Functions."Set Interface" ("Events"), error in (no error)=w677) -> (error out=w676:errorcluster)  [unwired: 1 in, 2 out]
      }
      event "Get Interface": Value Change {
        n300 = event-data() -> ()  [unwired: 1 in, 1 out]
        n301 = Enqueue Element(queue=w680, element=BiSS_Interface_Demo_Functions."Get Interface" ("Events"), error in (no error)=w682) -> (error out=w681:errorcluster)  [unwired: 1 in, 2 out]
      }
      event "Get Interface Info": Value Change {
        n302 = event-data() -> ()  [unwired: 1 in, 1 out]
        n303 = Enqueue Element(queue=w685, element=BiSS_Interface_Demo_Functions."Get Interface Info" ("Events"), error in (no error)=w687) -> (error out=w686:errorcluster)  [unwired: 1 in, 2 out]
      }
      event "Auto Detection": Value Change {
        n304 = event-data() -> ()  [unwired: 1 in, 1 out]
        n305 = Enqueue Element(queue=w690, element=BiSS_Interface_Demo_Functions."Auto Detection" ("Events"), error in (no error)=w691) -> (error out=w692:errorcluster)  [unwired: 1 in, 2 out]
      }
      event "Set Com Param": Value Change {
        n306 = event-data() -> ()  [unwired: 1 in, 1 out]
        n307 = Enqueue Element(queue=w695, element=BiSS_Interface_Demo_Functions."Set Com Param" ("Events"), error in (no error)=w697) -> (error out=w696:errorcluster)  [unwired: 1 in, 2 out]
      }
      event "Get Com Param": Value Change {
        n308 = event-data() -> ()  [unwired: 1 in, 1 out]
        n309 = Enqueue Element(queue=w700, element=BiSS_Interface_Demo_Functions."Get Com Param" ("Events"), error in (no error)=w702) -> (error out=w701:errorcluster)  [unwired: 1 in, 2 out]
      }
      event "Set Frame Param": Value Change {
        n310 = event-data() -> ()  [unwired: 1 in, 1 out]
        n311 = Enqueue Element(queue=w705, element=BiSS_Interface_Demo_Functions."Set Frame Param" ("Events"), error in (no error)=w706) -> (error out=w707:errorcluster)  [unwired: 1 in, 2 out]
      }
      event "Get Frame Param": Value Change {
        n312 = event-data() -> ()  [unwired: 1 in, 1 out]
        n313 = Enqueue Element(queue=w710, element=BiSS_Interface_Demo_Functions."Get Frame Param" ("Events"), error in (no error)=w712) -> (error out=w711:errorcluster)  [unwired: 1 in, 2 out]
      }
      event "Write Master Params": Value Change {
        n314 = event-data() -> ()  [unwired: 1 in, 1 out]
        n315 = Enqueue Element(queue=w715, element=BiSS_Interface_Demo_Functions."Write Master Params" ("Events"), error in (no error)=w717) -> (error out=w716:errorcluster)  [unwired: 1 in, 2 out]
      }
      event "Set FTDI Freq": Value Change {
        n316 = event-data() -> ()  [unwired: 1 in, 1 out]
        n317 = Enqueue Element(queue=w721, element=BiSS_Interface_Demo_Functions."Set FTDI Freq" ("Events"), error in (no error)=w722) -> (error out=w719:errorcluster)  [unwired: 1 in, 2 out]
      }
      event "Init BiSS Comm": Value Change {
        n318 = event-data() -> ()  [unwired: 1 in, 1 out]
        n319 = Enqueue Element(queue=w725, element=BiSS_Interface_Demo_Functions."Init BiSS Comm" ("Events"), error in (no error)=w727) -> (error out=w726:errorcluster)  [unwired: 1 in, 2 out]
      }
      event "Write Slave Register": Value Change {
        n320 = event-data() -> ()  [unwired: 1 in, 1 out]
        n321 = Enqueue Element(queue=w730, element=BiSS_Interface_Demo_Functions."Write Slave Register" ("Events"), error in (no error)=w732) -> (error out=w731:errorcluster)  [unwired: 1 in, 2 out]
      }
      event "Read Slave Register": Value Change {
        n322 = event-data() -> ()  [unwired: 1 in, 1 out]
        n323 = Enqueue Element(queue=w735, element=BiSS_Interface_Demo_Functions."Read Slave Register" ("Events"), error in (no error)=w737) -> (error out=w736:errorcluster)  [unwired: 1 in, 2 out]
      }
      event "Read SCD": Value Change {
        n324 = event-data() -> ()  [unwired: 1 in, 1 out]
        n325 = Enqueue Element(queue=w740, element=BiSS_Interface_Demo_Functions."Read SCD" ("Events"), error in (no error)=w742) -> (error out=w741:errorcluster)  [unwired: 1 in, 2 out]
      }
      event "Send Command": Value Change {
        n326 = event-data() -> ()  [unwired: 1 in, 1 out]
        n327 = Enqueue Element(queue=w745, element=BiSS_Interface_Demo_Functions."Send Command" ("Events"), error in (no error)=w747) -> (error out=w746:errorcluster)  [unwired: 1 in, 2 out]
      }
      event "Set Slave Label": Value Change {
        n328 = event-data() -> ()  [unwired: 1 in, 1 out]
        n329 = Enqueue Element(queue=w750, element=BiSS_Interface_Demo_Functions."Set Slave Label" ("Events"), error in (no error)=w752) -> (error out=w751:errorcluster)  [unwired: 1 in, 2 out]
      }
      event "Get Slave Label": Value Change {
        n330 = event-data() -> ()  [unwired: 1 in, 1 out]
        n331 = Enqueue Element(queue=w755, element=BiSS_Interface_Demo_Functions."Get Slave Label" ("Events"), error in (no error)=w757) -> (error out=w756:errorcluster)  [unwired: 1 in, 2 out]
      }
      event "Set SCD Content Labels": Value Change {
        n332 = event-data() -> ()  [unwired: 1 in, 1 out]
        n333 = Enqueue Element(queue=w760, element=BiSS_Interface_Demo_Functions."Set SCD Content Labels" ("Events"), error in (no error)=w762) -> (error out=w761:errorcluster)  [unwired: 1 in, 2 out]
      }
      event "Get SCD Content Labels": Value Change {
        n334 = event-data() -> ()  [unwired: 1 in, 1 out]
        n335 = Enqueue Element(queue=w765, element=BiSS_Interface_Demo_Functions."Get SCD Content Labels" ("Events"), error in (no error)=w767) -> (error out=w766:errorcluster)  [unwired: 1 in, 2 out]
      }
      event "Get SCD Content": Value Change {
        n336 = event-data() -> ()  [unwired: 1 in, 1 out]
        n337 = Enqueue Element(queue=w771, element=BiSS_Interface_Demo_Functions."Get SCD Content" ("Events"), error in (no error)=w772) -> (error out=w770:errorcluster)  [unwired: 1 in, 2 out]
      }
      event "Get SCD Content Ex": Value Change {
        n338 = event-data() -> ()  [unwired: 1 in, 1 out]
        n339 = Enqueue Element(queue=w774, element=BiSS_Interface_Demo_Functions."Get SCD Content Ex" ("Events"), error in (no error)=w775) -> (error out=w773:errorcluster)  [unwired: 1 in, 2 out]
      }
      event "Set SCD Content Params": Value Change {
        n340 = event-data() -> ()  [unwired: 1 in, 1 out]
        n341 = Enqueue Element(queue=w779, element=BiSS_Interface_Demo_Functions."Set SCD Content Params" ("Events"), error in (no error)=w780) -> (error out=w778:errorcluster)  [unwired: 1 in, 2 out]
      }
      event "Get SCD Content Params": Value Change {
        n342 = event-data() -> ()  [unwired: 1 in, 1 out]
        n343 = Enqueue Element(queue=w784, element=BiSS_Interface_Demo_Functions."Get SCD Content Params" ("Events"), error in (no error)=w785) -> (error out=w783:errorcluster)  [unwired: 1 in, 2 out]
      }
      event "Read SCD Frames": Value Change {
        n344 = event-data() -> ()  [unwired: 1 in, 1 out]
        n345 = Enqueue Element(queue=w789, element=BiSS_Interface_Demo_Functions."Read SCD Frames" ("Events"), error in (no error)=w790) -> (error out=w788:errorcluster)  [unwired: 1 in, 2 out]
      }
      event "Get SCD Frame": Value Change {
        n346 = event-data() -> ()  [unwired: 1 in, 1 out]
        n347 = Enqueue Element(queue=w794, element=BiSS_Interface_Demo_Functions."Get SCD Frame" ("Events"), error in (no error)=w795) -> (error out=w793:errorcluster)  [unwired: 1 in, 2 out]
      }
      event "Get SCD Frame Ex": Value Change {
        n348 = event-data() -> ()  [unwired: 1 in, 1 out]
        n349 = Enqueue Element(queue=w799, element=BiSS_Interface_Demo_Functions."Get SCD Frame Ex" ("Events"), error in (no error)=w800) -> (error out=w798:errorcluster)  [unwired: 1 in, 2 out]
      }
      event "Get SCD Frame Content": Value Change {
        n350 = event-data() -> ()  [unwired: 1 in, 1 out]
        n351 = Enqueue Element(queue=w804, element=BiSS_Interface_Demo_Functions."Get SCD Frame Content" ("Events"), error in (no error)=w805) -> (error out=w803:errorcluster)  [unwired: 1 in, 2 out]
      }
      event "Get SCD Frame Content Ex": Value Change {
        n352 = event-data() -> ()  [unwired: 1 in, 1 out]
        n353 = Enqueue Element(queue=w809, element=BiSS_Interface_Demo_Functions."Get SCD Frame Content Ex", error in (no error)=w811) -> (error out=w810:errorcluster)  [unwired: 1 in, 2 out]
      }
      event "Get EDS Param": Value Change {
        n354 = event-data() -> ()  [unwired: 1 in, 1 out]
        n355 = Enqueue Element(queue=w814, element=BiSS_Interface_Demo_Functions."Get EDS Param" ("Events"), error in (no error)=w815) -> (error out=w813:errorcluster)  [unwired: 1 in, 2 out]
      }
      event "Set EDS Param": Value Change {
        n356 = event-data() -> ()  [unwired: 1 in, 1 out]
        n357 = Enqueue Element(queue=w819, element=BiSS_Interface_Demo_Functions."Set EDS Param" ("Events"), error in (no error)=w820) -> (error out=w818:errorcluster)  [unwired: 1 in, 2 out]
      }
      event "Set EDS Register": Value Change {
        n358 = event-data() -> ()  [unwired: 1 in, 1 out]
        n359 = Enqueue Element(queue=w824, element=BiSS_Interface_Demo_Functions."Set EDS Register" ("Events"), error in (no error)=w825) -> (error out=w823:errorcluster)  [unwired: 1 in, 2 out]
      }
      event "Get EDS Register": Value Change {
        n360 = event-data() -> ()  [unwired: 1 in, 1 out]
        n361 = Enqueue Element(queue=w829, element=BiSS_Interface_Demo_Functions."Get EDS Register" ("Events"), error in (no error)=w830) -> (error out=w828:errorcluster)  [unwired: 1 in, 2 out]
      }
      event "Read EDS Params": Value Change {
        n362 = event-data() -> ()  [unwired: 1 in, 1 out]
        n363 = Enqueue Element(queue=w834, element=BiSS_Interface_Demo_Functions."Read EDS Params" ("Events"), error in (no error)=w835) -> (error out=w833:errorcluster)  [unwired: 1 in, 2 out]
      }
      event "Write EDS Params": Value Change {
        n364 = event-data() -> ()  [unwired: 1 in, 1 out]
        n365 = Enqueue Element(queue=w839, element=BiSS_Interface_Demo_Functions."Write EDS Params" ("Events"), error in (no error)=w840) -> (error out=w838:errorcluster)  [unwired: 1 in, 2 out]
      }
      event "Get DLL Version": Value Change {
        n366 = event-data() -> ()  [unwired: 1 in, 1 out]
        n367 = Enqueue Element(queue=w844, element=BiSS_Interface_Demo_Functions."Get DLL Version" ("Events"), error in (no error)=w845) -> (error out=w843:errorcluster)  [unwired: 1 in, 2 out]
      }
      event "Calculate CRC": Value Change {
        n368 = event-data() -> ()  [unwired: 1 in, 1 out]
        n369 = Enqueue Element(queue=w849, element=BiSS_Interface_Demo_Functions."Calculate CRC" ("Events"), error in (no error)=w850) -> (error out=w848:errorcluster)  [unwired: 1 in, 2 out]
      }
      event "Calculate CRC Ex": Value Change {
        n370 = event-data() -> ()  [unwired: 1 in, 1 out]
        n371 = Enqueue Element(queue=w854, element=BiSS_Interface_Demo_Functions."Calculate CRC Ex" ("Events"), error in (no error)=w855) -> (error out=w853:errorcluster)  [unwired: 1 in, 2 out]
      }
      event "Save DLL Config": Value Change {
        n372 = event-data() -> ()  [unwired: 1 in, 1 out]
        n373 = Enqueue Element(queue=w859, element=BiSS_Interface_Demo_Functions."Save DLL Config" ("Events"), error in (no error)=w860) -> (error out=w858:errorcluster)  [unwired: 1 in, 2 out]
      }
      event "Load DLL Config": Value Change {
        n374 = event-data() -> ()  [unwired: 1 in, 1 out]
        n375 = Enqueue Element(queue=w864, element=BiSS_Interface_Demo_Functions."Load DLL Config" ("Events"), error in (no error)=w865) -> (error out=w863:errorcluster)  [unwired: 1 in, 2 out]
      }
      event "Get Last Error": Value Change {
        n376 = event-data() -> ()  [unwired: 1 in, 1 out]
        n377 = Enqueue Element(queue=w869, element=BiSS_Interface_Demo_Functions."Get Last Error" ("Events"), error in (no error)=w870) -> (error out=w868:errorcluster)  [unwired: 1 in, 2 out]
      }
      event "Get MB3U Pins": Value Change {
        n378 = event-data() -> ()  [unwired: 1 in, 1 out]
        n379 = Enqueue Element(queue=w874, element=BiSS_Interface_Demo_Functions."Get MB3U Pins" ("Events"), error in (no error)=w875) -> (error out=w873:errorcluster)  [unwired: 1 in, 2 out]
      }
      event "Set MB3U Pins": Value Change {
        n380 = event-data() -> ()  [unwired: 1 in, 1 out]
        n381 = Enqueue Element(queue=w879, element=BiSS_Interface_Demo_Functions."Set MB3U Pins" ("Events"), error in (no error)=w880) -> (error out=w878:errorcluster)  [unwired: 1 in, 2 out]
      }
      event "Write Master Register": Value Change {
        n382 = event-data() -> ()  [unwired: 1 in, 1 out]
        n383 = Enqueue Element(queue=w884, element=BiSS_Interface_Demo_Functions."Write Master Register" ("Events"), error in (no error)=w885) -> (error out=w883:errorcluster)  [unwired: 1 in, 2 out]
      }
      event "Read Master Register": Value Change {
        n384 = event-data() -> ()  [unwired: 1 in, 1 out]
        n385 = Enqueue Element(queue=w889, element=BiSS_Interface_Demo_Functions."Read Master Register" ("Events"), error in (no error)=w890) -> (error out=w888:errorcluster)  [unwired: 1 in, 2 out]
      }
      event "Get Master Register": Value Change {
        n386 = event-data() -> ()  [unwired: 1 in, 1 out]
        n387 = Enqueue Element(queue=w894, element=BiSS_Interface_Demo_Functions."Get Master Register" ("Events"), error in (no error)=w895) -> (error out=w893:errorcluster)  [unwired: 1 in, 2 out]
      }
      event "Save Master Config": Value Change {
        n388 = event-data() -> ()  [unwired: 1 in, 1 out]
        n389 = Enqueue Element(queue=w899, element=BiSS_Interface_Demo_Functions."Save Master Config" ("Events"), error in (no error)=w900) -> (error out=w898:errorcluster)  [unwired: 1 in, 2 out]
      }
      event "Save Register": Value Change {
        n390 = event-data() -> ()  [unwired: 1 in, 1 out]
        n391 = Enqueue Element(queue=w904, element=BiSS_Interface_Demo_Functions."Save Register" ("Events"), error in (no error)=w905) -> (error out=w903:errorcluster)  [unwired: 1 in, 2 out]
      }
      event "Load Register": Value Change {
        n392 = event-data() -> ()  [unwired: 1 in, 1 out]
        n393 = Enqueue Element(queue=w909, element=BiSS_Interface_Demo_Functions."Load Register" ("Events"), error in (no error)=w910) -> (error out=w908:errorcluster)  [unwired: 1 in, 2 out]
      }
      event "Stop Button": Value Change {
        n394 = event-data() -> ()  [unwired: 1 in, 1 out]
        n395 = Enqueue Element At Opposite End(queue=w915, element=BiSS_Interface_Demo_Functions."Stop Demo" ("Events"), error in (no error)=w916) -> (error out=w914:errorcluster)  [unwired: 1 in, 2 out]
      }
    }
    n396 = call <vilib>:"Simple Error Handler.vi"("error in (no error)"=w660) -> ()  [unwired: 4 in, 5 out]
  }
